vi "Confocal_Ver3.12f - sm correction.vi"() -> ()   [LabVIEW 2009]
uses:
  <vilib>/DAQmx/configure/timing.llb/DAQmx Timing (Sample Clock).vi
  <vilib>/DAQmx/create/channels.llb/DAQmx Create Channel (AI-Voltage-Basic).vi
  <vilib>/DAQmx/create/channels.llb/DAQmx Create Channel (AO-Voltage-Basic).vi
  <vilib>/DAQmx/write.llb/DAQmx Write (Analog 2D DBL NChan NSamp).vi
  <vilib>/DAQmx/read.llb/DAQmx Read (Analog 1D DBL NChan 1Samp).vi
  <vilib>/DAQmx/configure/trigger.llb/DAQmx Start Trigger (Digital Edge).vi
  <vilib>/DAQmx/read.llb/DAQmx Read (Analog 2D DBL NChan NSamp).vi
  <vilib>/DAQmx/write.llb/DAQmx Write (Analog 1D DBL NChan 1Samp).vi
  <vilib>/measure/NI_MABase.lvlib
  Program Files (x86)/National Instruments/LabVIEW 2009/resource/objmgr/daqmx.rc
panel:
  in  "Volts/pixel":dbl=0.1
  in  "Correction":dbl[][](array[numeric])=[[600.0, 650.0, 10.0, 5.0]]
  in  "sm correction?":bool
  out "Boolean":bool
  in  "Update":bool
  in  "StopPoint":dbl
  in  "Concat":bool
  in  "Increment":bool
  in  "stepsize":dbl=0.001
  in  "y 2":cluster{dbl, string, tag}[](array[cluster])=[{1.0, "", "Dev1/ai19"}, {1.0, "", "Dev1/ai16"}, {1.0, "", ""}, {1.0, "", ""}, {0.0, "", ""}, {1.0, "", ""}]
  in  "y":cluster{dbl, string, tag}[](array[cluster])=[{1.0, "", "Dev1/ao1"}, {1.0, "", "Dev1/ao0"}, {1.0, "", "Dev1/ao2"}, {1.0, "", "Dev1/ao3"}, {0.0, "", ""}, {1.0, "", ""}]
  in  "?":bool
  in  "Output4":dbl min=-10.0 max=10.0 step=0.1
  in  "Output3":dbl min=-10.0 max=10.0 step=0.1
  in  "Starting Point for Scan":tag="Dev1/ai1:2"
  in  "output scale":i32=1
  in  "out/in":dbl=1.0
  in  "Channel 2":path=path "T:/Physics/Minot Group/Lee/SPCM/2013-8-22/surf36_20"
  in  "Channel 1":path=path "T:/Physics/Minot Group/Lee/SPCM/2013-8-22/surf36_20"
  in  "Save Image":bool
  out "Channel2":dbl[][](graph)
  in  "Scanner delay (ms)":dbl=0.16
  in  "Lines read":u32=1
  out "Reflection Image":dbl[][](graph)
  out "Linescan":dbl[][](graph)=[[0.48392498883474516, 0.48650485009910055, 0.4823125755469766, 0.48553740212440066, 0.4842474714925252, 0.4852149194663185, 0.48392498883474516, 0.48263505820437946, 0.4813451275752202, 0.4813451275752202, 0.4813451275752202, 0.4787652663205165, 0.4823125755469766, 0.4748954744474811, 0.47650788772659863, 0.47586292241472655, 0.47618540507062507, 0.47586292241472655, 0.47715285303877103, 0.479732714290466, 0.4829575408618577, 0.48392498883474516, 0.48392498883474516, 0.4861823674407917, 0.48585988478255837, 0.4884397460505425, 0.4884397460505425, 0.48553740212440066, 0.48747229807448106, 0.4903746420047106, 0.4903746420047106, 0.4900521593454931, 0.4900521593454931, 0.4881172633917797, 0.4861823674407917, 0.4884397460505425, 0.4903746420047106, 0.4884397460505425, 0.4897296766863515, 0.4881172633917797, 0.48650485009910055, 0.48876222870938113, 0.4890847113682955, 0.4842474714925252, 0.4842474714925252, 0.4823125755469766, 0.4842474714925252, 0.4845699541503808, 0.4790877489770911, 0.4813451275752202, 0.479732714290466, 0.48070016226109263, 0.4800551969472663, 0.4784427836640171, 0.4803776796041418, 0.48166761023239696, 0.4832800235194114, 0.48166761023239696, 0.48102264491811875, 0.4852149194663185, 0.48650485009910055, 0.48585988478255837, 0.4877947807330925, 0.4871498154159452, 0.4894071940272856, 0.4881172633917797, 0.4871498154159452, 0.4900521593454931, 0.4877947807330925, 0.48747229807448106, 0.4861823674407917, 0.4848924368083119, 0.4832800235194114, 0.4871498154159452, 0.4871498154159452, 0.48553740212440066, 0.4868273327574851, 0.4852149194663185, 0.4852149194663185, 0.48263505820437946, 0.48166761023239696, 0.4800551969472663, 0.48102264491811875, 0.48392498883474516, 0.48070016226109263, 0.4787652663205165, 0.4748954744474811, 0.47457299179188256, 0.47296057851501405, 0.4736055438255367, 0.4703807172759168, 0.47747533569496986, 0.4842474714925252, 0.4997266391550764, 0.5158507723239795, 0.5342322843721873, 0.544229247171595, 0.573252687987951, 0.591634200841002, 0.6087257832047819, 0.6219475734938213, 0.6325895023644409, 0.6422639832349691, 0.6493586025881635, 0.6567757046830137, 0.6629028760126687, 0.6632253587150819, 0.6606454970981651, 0.6632253587150819, 0.6635478414175805, 0.6612904625018826, 0.6590330835903624, 0.6635478414175805, 0.6612904625018826, 0.6612904625018826, 0.6619354279059412, 0.6535508776797399, 0.6541958430797155, 0.650648533384047, 0.6516159814818486, 0.650648533384047, 0.6512934987824968, 0.6522609468808066, 0.6535508776797399, 0.6529059122801036, 0.6503260506849492, 0.6503260506849492, 0.6480686717936336, 0.6458112929064599, 0.6471012236986238, 0.6454888102086299, 0.6422639832349691, 0.6445213621156465, 0.6471012236986238, 0.6480686717936336, 0.650003567985936, 0.6535508776797399, 0.6545183257798305, 0.6538733603796852, 0.6535508776797399, 0.6551632911803154, 0.6561307392816795, 0.6600005316947886, 0.6622579106080984, 0.6587106008890573, 0.6606454970981651, 0.6577431527856528, 0.6587106008890573, 0.6580656354867026, 0.659678048993228, 0.6561307392816795, 0.6590330835903624, 0.6577431527856528, 0.6525834295804127, 0.6567757046830137, 0.6480686717936336, 0.6451663275108844, 0.6429089486290271, 0.6364592947035884, 0.6338794331428164, 0.6280747446506622, 0.6267848138783022, 0.6274297792643154, 0.6303321235055045, 0.6319445369757553, 0.63710426009462, 0.6387166735736678, 0.6409740524478638, 0.6474237063968759, 0.6496810852870074, 0.6532283949798794, 0.6529059122801036, 0.6529059122801036, 0.6538733603796852, 0.6538733603796852, 0.6541958430797155, 0.6545183257798305, 0.6554857738806851, 0.6570981873838084, 0.6593555662917526, 0.6606454970981651, 0.6616129452038693, 0.6658052203374621, 0.6632253587150819, 0.6616129452038693, 0.6622579106080984, 0.6645152895255886, 0.6570981873838084, 0.6567757046830137, 0.6525834295804127, 0.6483911544921392, 0.650648533384047, 0.6480686717936336, 0.6454888102086299, 0.6467787410004561, 0.6438763967207458, 0.6477461890952124, 0.650648533384047, 0.6461337756043742, 0.6512934987824968], [-0.0030237485169774024, -0.0030237485169774024, -0.0030237485169774024, -0.0030237485169774024, -0.003346231081005397, -0.0020563008246016422, -0.0036687136449847922, -0.0030237485169774024, -0.003346231081005397, -0.0030237485169774024, -0.0036687136449847922, -0.003346231081005397, -0.0030237485169774024, -0.00270126595290079, -0.0023787833887755428, -0.0036687136449847922, -0.003346231081005397, -0.0036687136449847922, -0.0036687136449847922, -0.003346231081005397, -0.003346231081005397, -0.0030237485169774024, -0.0036687136449847922, -0.0036687136449847922, -0.004313678772797855, -0.003991196208915606, -0.0030237485169774024, -0.0030237485169774024, -0.0036687136449847922, -0.003346231081005397, -0.003991196208915606, -0.0030237485169774024, -0.0030237485169774024, -0.003346231081005397, -0.003346231081005397, -0.0020563008246016422, -0.00270126595290079, -0.0020563008246016422, -0.0020563008246016422, -0.0020563008246016422, -0.0030237485169774024, -0.00270126595290079, -0.003346231081005397, -0.00270126595290079, -0.0030237485169774024, -0.0036687136449847922, -0.0036687136449847922, -0.003991196208915606, -0.0030237485169774024, -0.0036687136449847922, -0.0023787833887755428, -0.0030237485169774024, -0.00270126595290079, -0.003346231081005397, -0.00270126595290079, -0.00270126595290079, -0.0030237485169774024, -0.00270126595290079, -0.003991196208915606, -0.0036687136449847922, -0.003346231081005397, -0.0030237485169774024, -0.003991196208915606, -0.003346231081005397, -0.0036687136449847922, -0.003346231081005397, -0.00270126595290079, -0.0036687136449847922, -0.0030237485169774024, -0.0036687136449847922, -0.003346231081005397, -0.003346231081005397, -0.0036687136449847922, -0.003991196208915606, -0.0036687136449847922, -0.0036687136449847922, -0.003346231081005397, -0.0036687136449847922, -0.0036687136449847922, -0.003991196208915606, -0.0036687136449847922, -0.0030237485169774024, -0.0036687136449847922, -0.00270126595290079, -0.004313678772797855, -0.004958643900416732, -0.0065710567186153, -0.0068935392821096765, -0.008505952098855858, -0.008828434662060078, -0.010118364914394162, -0.01108581260313829, -0.010440847477357074, -0.008183469535603323, -0.005603609027841567, -0.00270126595290079, 0.0014910073845274476, 0.00858562382054782, 0.013422862313310125, 0.018905065951914643, 0.022774856764300203, 0.027289612721192864, 0.030836920979949438, 0.03180436868794224, 0.03277181639638989, 0.03277181639638989, 0.03180436868794224, 0.030836920979949438, 0.02890202556532645, 0.026322165015316323, 0.024709752173193242, 0.02180740906052947, 0.02051747878953489, 0.019227548519338968, 0.016647687981338526, 0.01568024028040894, 0.014712792579926194, 0.01277789718029931, 0.01277789718029931, 0.011487966914871401, 0.00955307151821172, 0.00858562382054782, 0.007940658689018203, 0.006973210992092902, 0.00600576329561012, 0.006328245861055242, 0.005683280730214114, 0.005360798164867205, 0.005038315599569377, 0.004070867903970193, 0.00471583303432061, 0.004070867903970193, 0.0031034202088120865, 0.0027809376438573193, 0.0018134899492865714, 0.0014910073845274476, 0.0014910073845274476, 0.0021359725140945793, 0.0014910073845274476, 0.0008460422551557815, 0.00020107712597943893, 0.0005235596905432037, -0.0004438880030017225, -0.0004438880030017225, -0.0004438880030017225, -0.0007663705674191548, -0.0007663705674191548, -0.001088853131787845, -0.0014113356961078113, -0.001733818260379071, -0.0023787833887755428, -0.001733818260379071, -0.0023787833887755428, -0.001733818260379071, -0.0023787833887755428, -0.0023787833887755428, -0.0020563008246016422, -0.00270126595290079, -0.0023787833887755428, -0.0020563008246016422, -0.00270126595290079, -0.00270126595290079, -0.0023787833887755428, -0.001733818260379071, -0.0014113356961078113, -0.001733818260379071, -0.0023787833887755428, -0.0023787833887755428, -0.0023787833887755428, -0.0023787833887755428, -0.00270126595290079, -0.0020563008246016422, -0.003346231081005397, -0.0023787833887755428, -0.00270126595290079, -0.00270126595290079, -0.0020563008246016422, -0.0030237485169774024, -0.0023787833887755428, -0.0030237485169774024, -0.0020563008246016422, -0.003346231081005397, -0.0023787833887755428, -0.00270126595290079, -0.0030237485169774024, -0.0020563008246016422, -0.003346231081005397, -0.003346231081005397, -0.003991196208915606, -0.003346231081005397, -0.00270126595290079, -0.0030237485169774024, -0.0036687136449847922, -0.00270126595290079, -0.0023787833887755428, -0.00270126595290079, -0.003991196208915606, -0.0036687136449847922, -0.003346231081005397, -0.00270126595290079]]
  out "Output rate":dbl=31250.0
  out "Input rate":dbl=31250.0
  in  "Y Scan size(um)":dbl=2.0
  in  "Reset":bool
  in  "Stop":bool
  in  "Continuous \nScan":bool=TRUE
  in  "Finite scan":bool
  in  "Conversion \n(mV/um)":dbl=41.0
  in  "Scan Lines":u32=200
  in  "Scan Points":u32=200
  in  "Scan Angle (degrees)":dbl
  in  "X offset (um)":dbl=-0.4599999999999997
  in  "Y offset (um)":dbl=-0.23
  in  "Scan Rate (Hz)":dbl=25.0
  in  "X Scan size(um)":dbl=2.0
  in  "minimum value":dbl=-4.0 caption="Output Minimum Value" format="%0.2f"
  in  "maximum value":dbl=4.0 caption="Output Maximum Value" format="%0.2f"
  in  "Maximum Value":dbl=10.0 caption="Input Maximum Value" format="%0.2f"
  in  "Minimum Value":dbl=-10.0 caption="Input Minimum Value" format="%0.2f"
  # "Scan channel 1"
  # "Scan channel 2"
  # "Device"
  # "Output channel 3"
  # "Output channel 4"
  # "Input channel 1"
  # "Input channel 2"
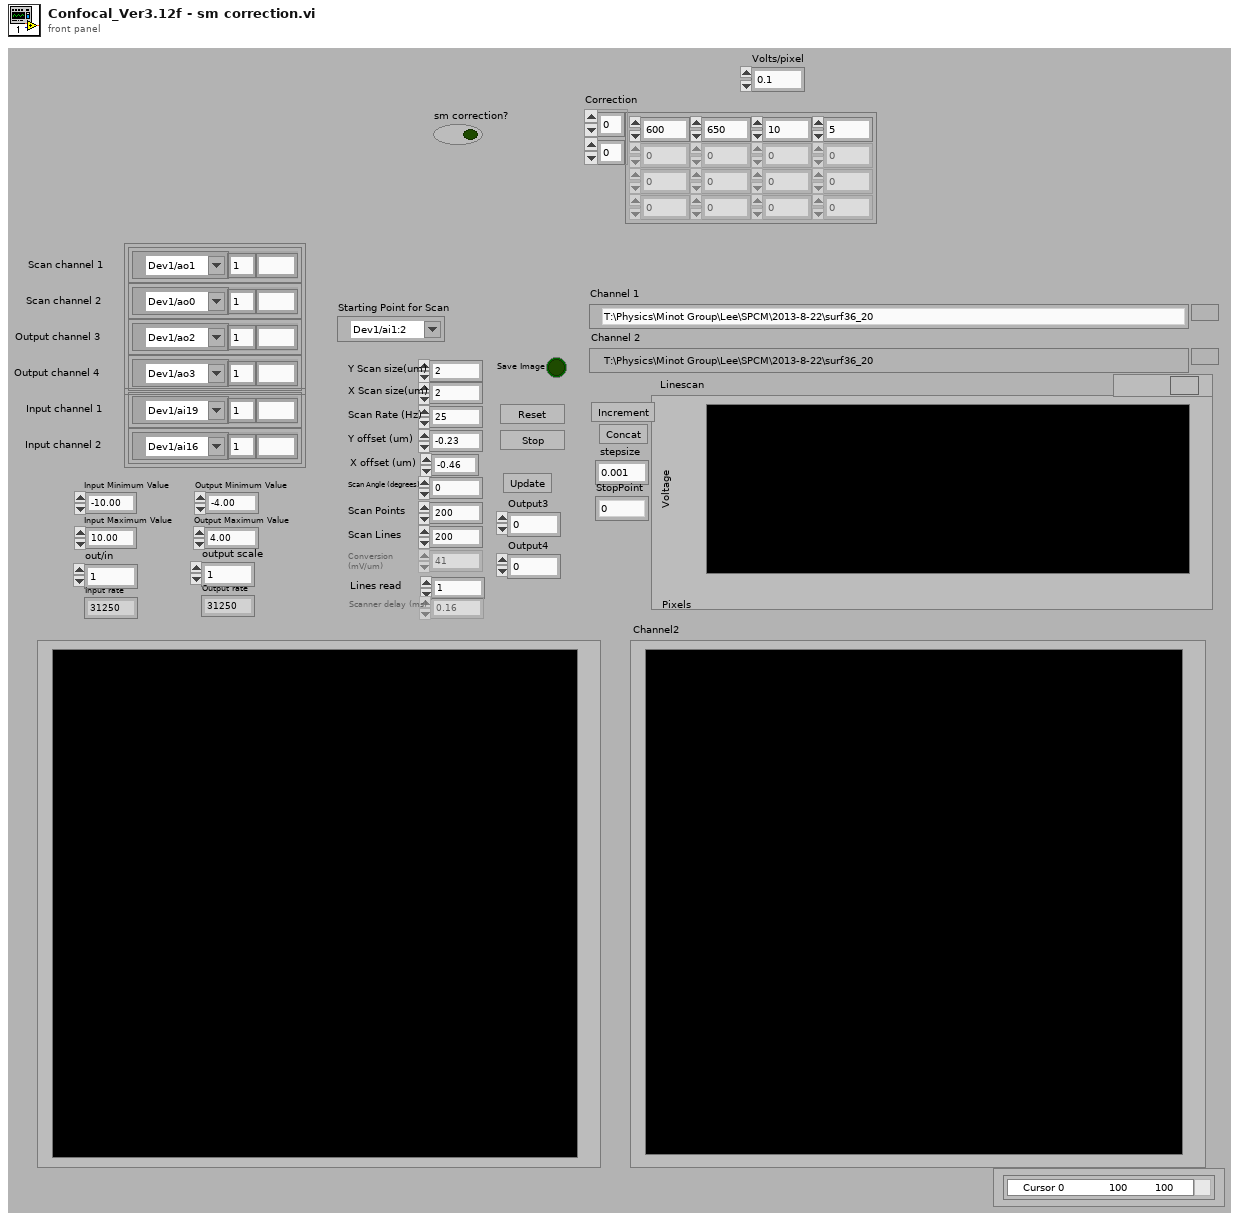
[diagram p1: front panel]
types:
  T1 = enum16{"Sine Wave", "Triangle Wave", "Square Wave", "Sawtooth Wave"}
  T2 = cluster{"Y Scan size(um) ":dbl, "X Scan size(um)":dbl, "Scan Rate (Hz)":dbl, "Y offset (um)":dbl, "X offset (um)":dbl, "Scan Angle (degrees)":dbl, "Scan Points":u32, "Scan Lines":u32, "Conversion \n(mV/um)":dbl, "Finite scan":bool, "Continuous \nScan":bool, "Lines read":u32, "Scanner delay (ms)":dbl}
  T3 = enum16{"open", "open or create", "create or replace", "create", "open (read only)"}
  T4 = typedef "LVPointDoubleTypeDef.ctl" = cluster{"Cursor X":dbl, "Cursor Y":dbl}
  T5 = cluster{"X offset (um)":dbl, "Y offset (um)":dbl}
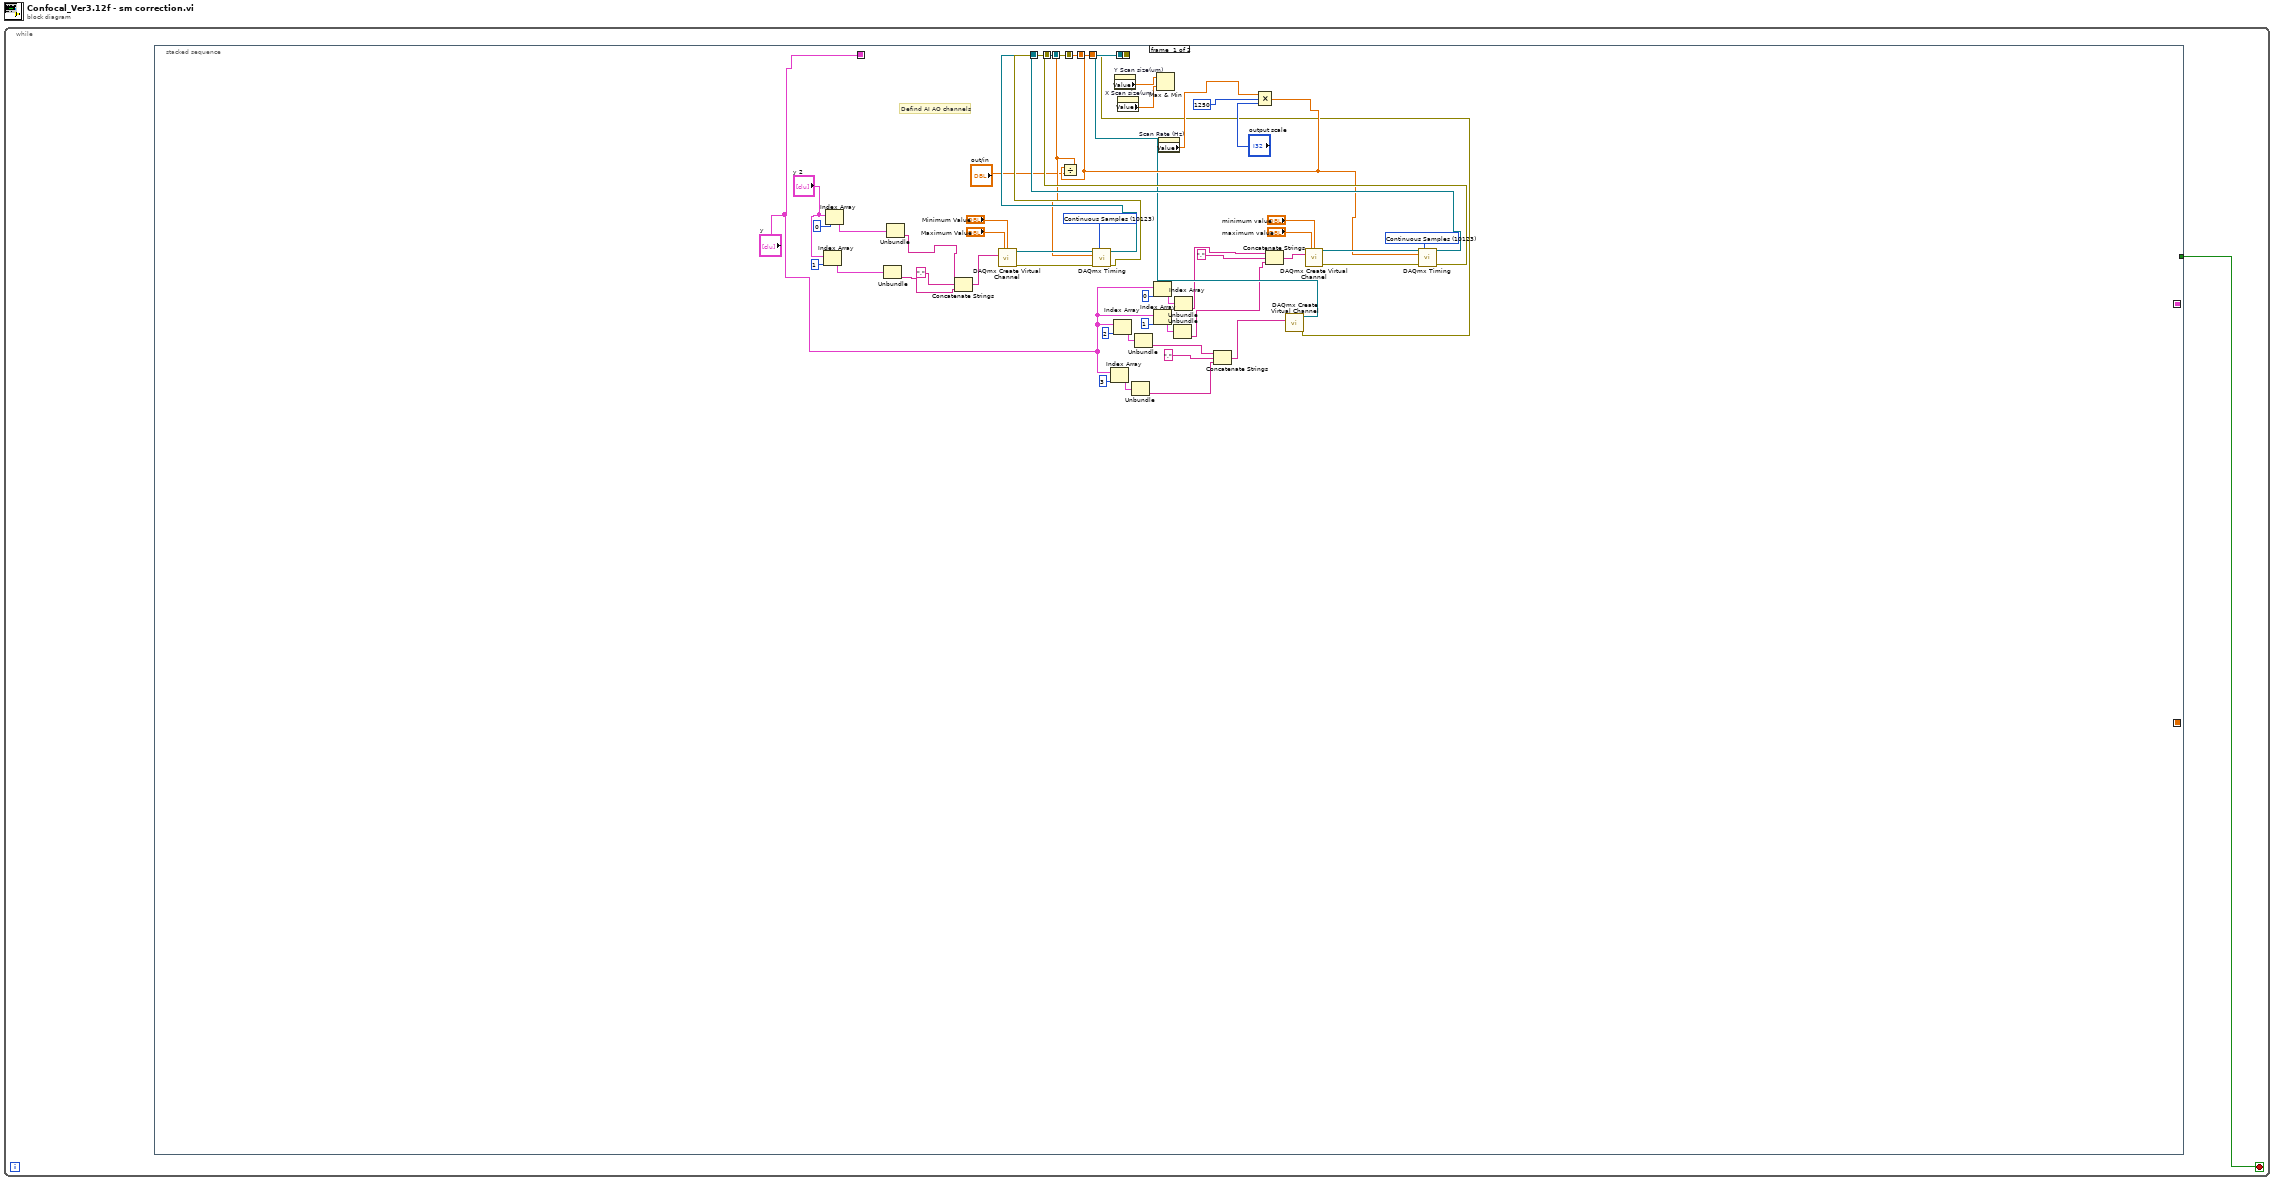
[diagram p0: block diagram]
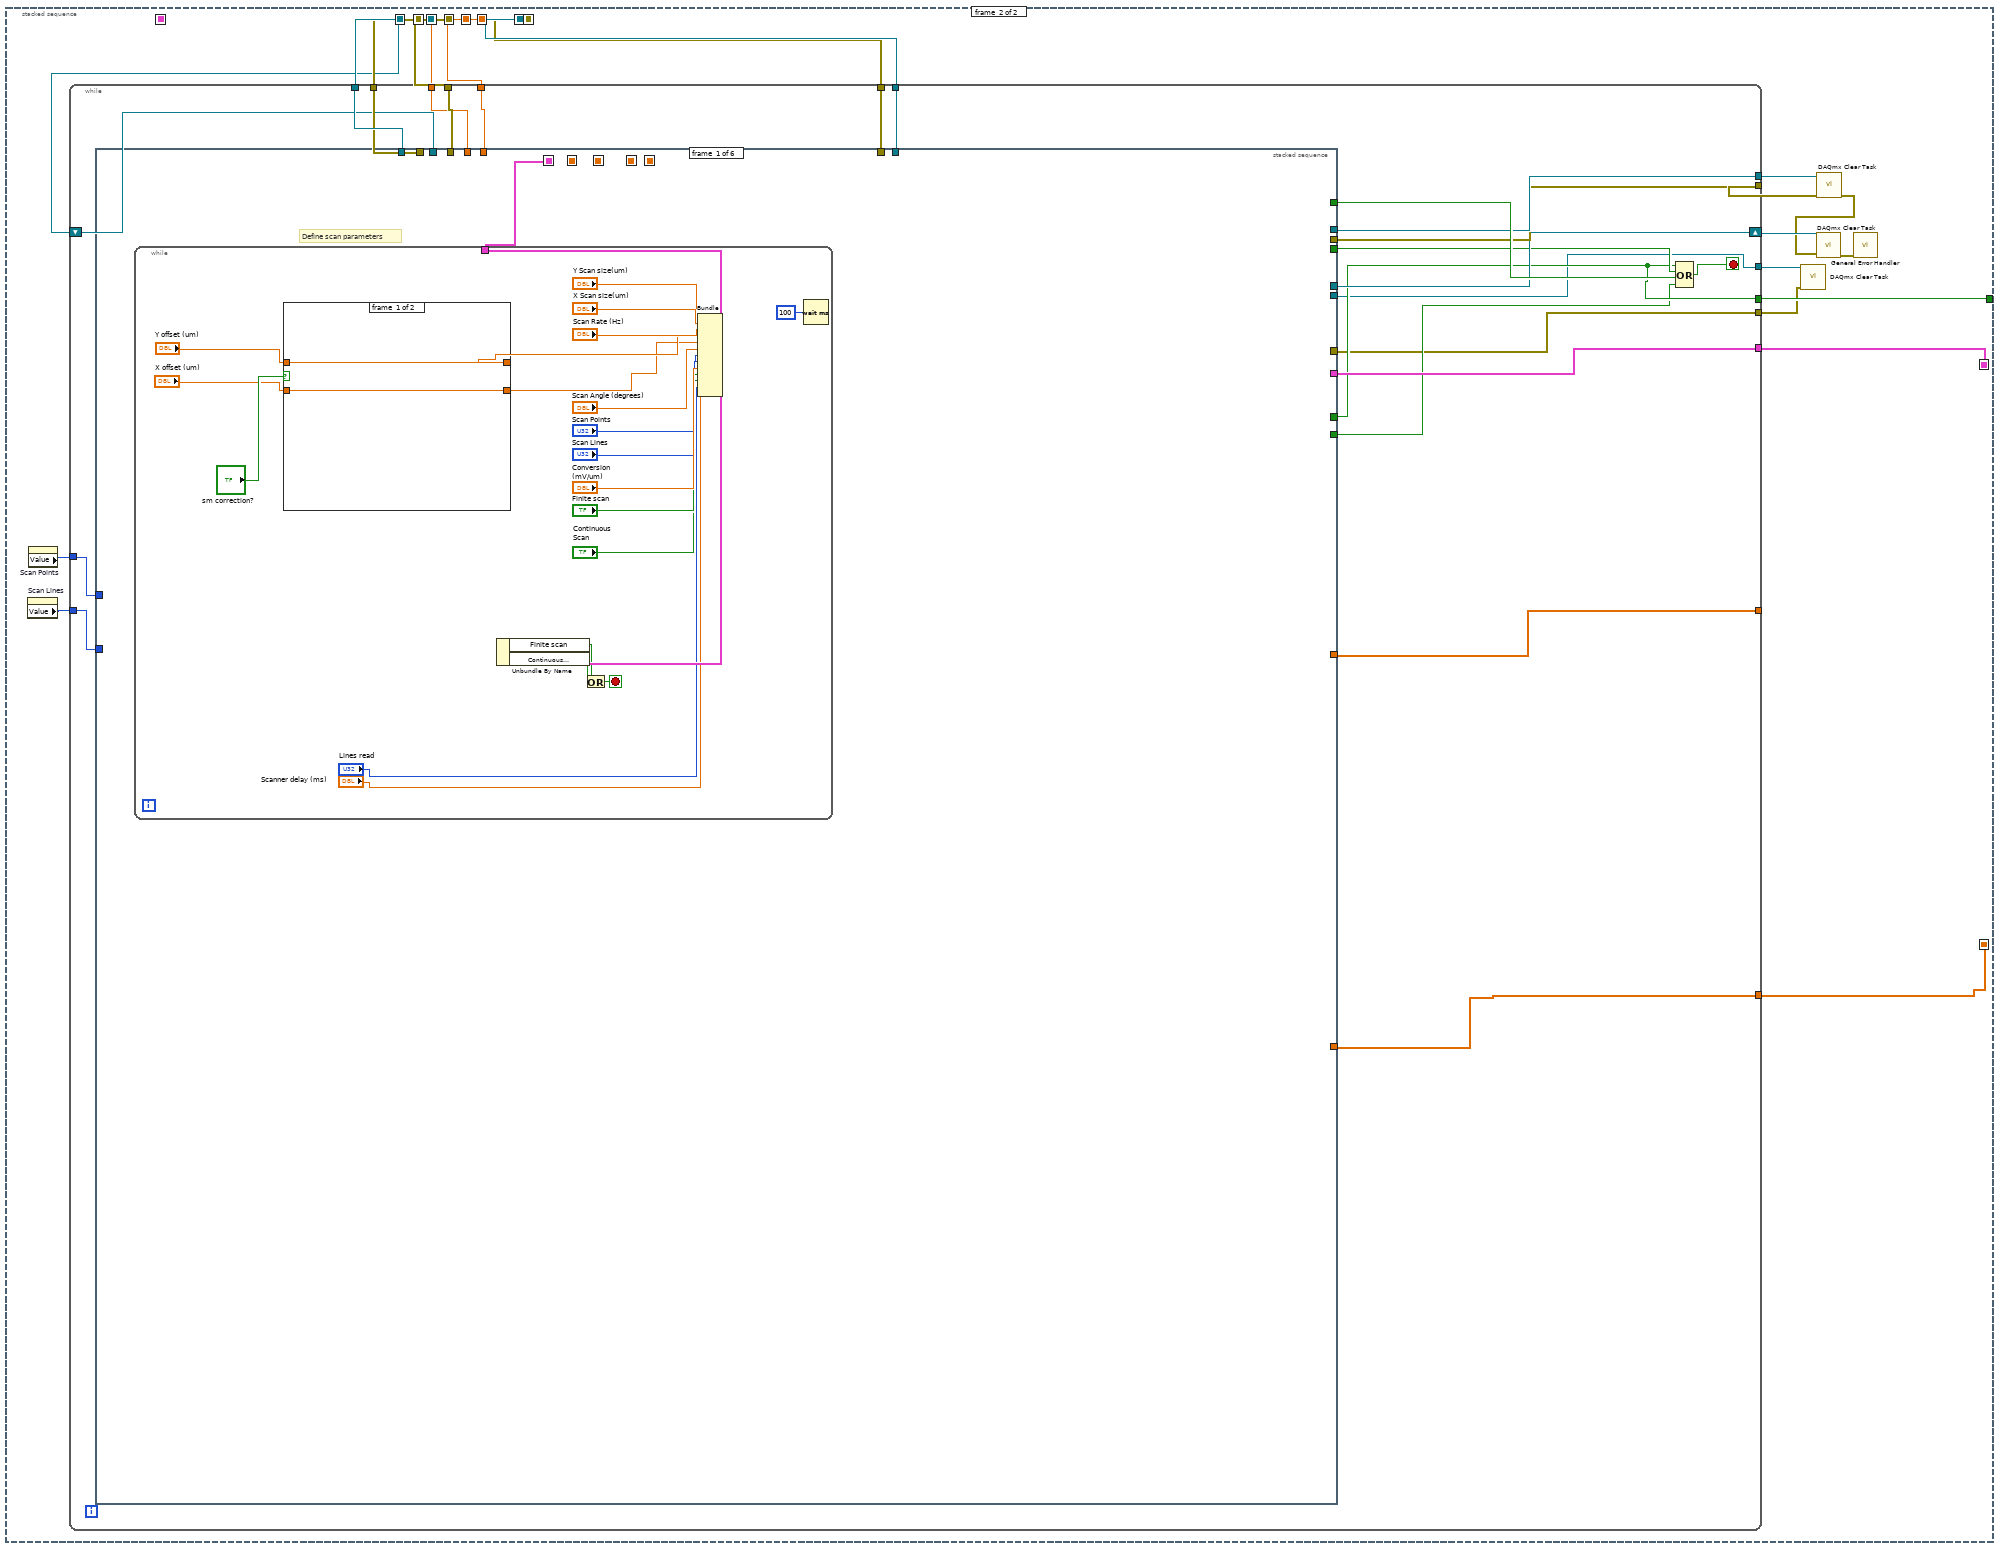
[diagram p2: hidden frame]
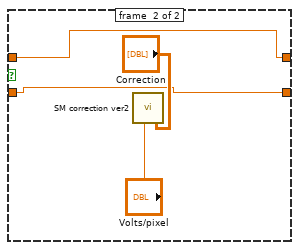
[diagram p3: hidden frame]
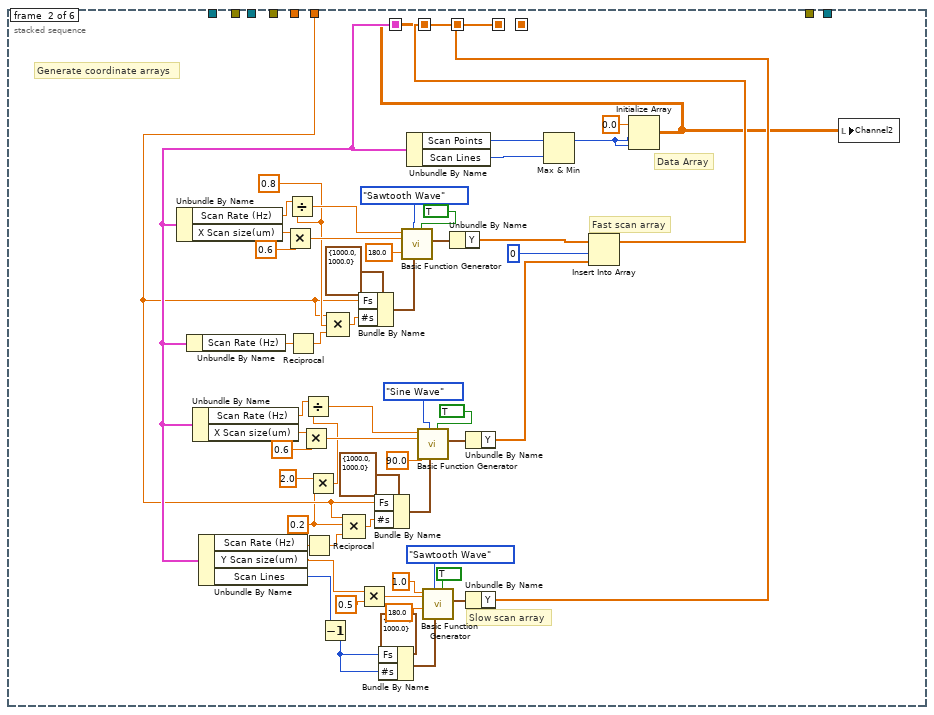
[diagram p4: hidden frame]
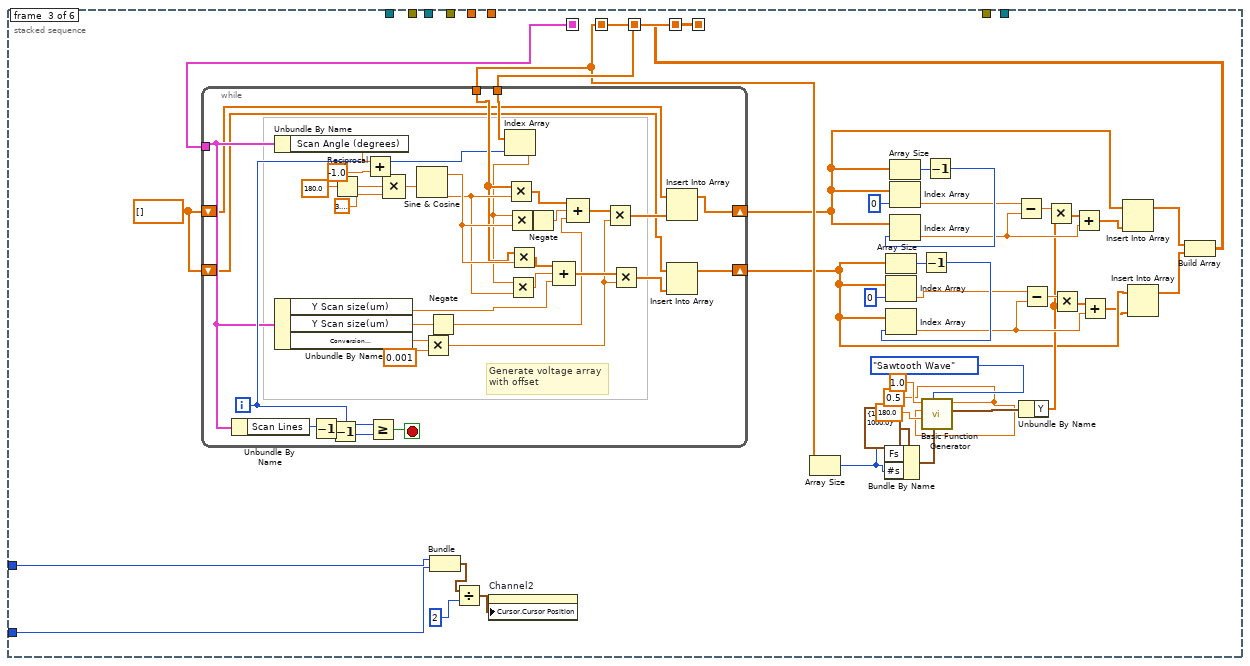
[diagram p5: hidden frame]
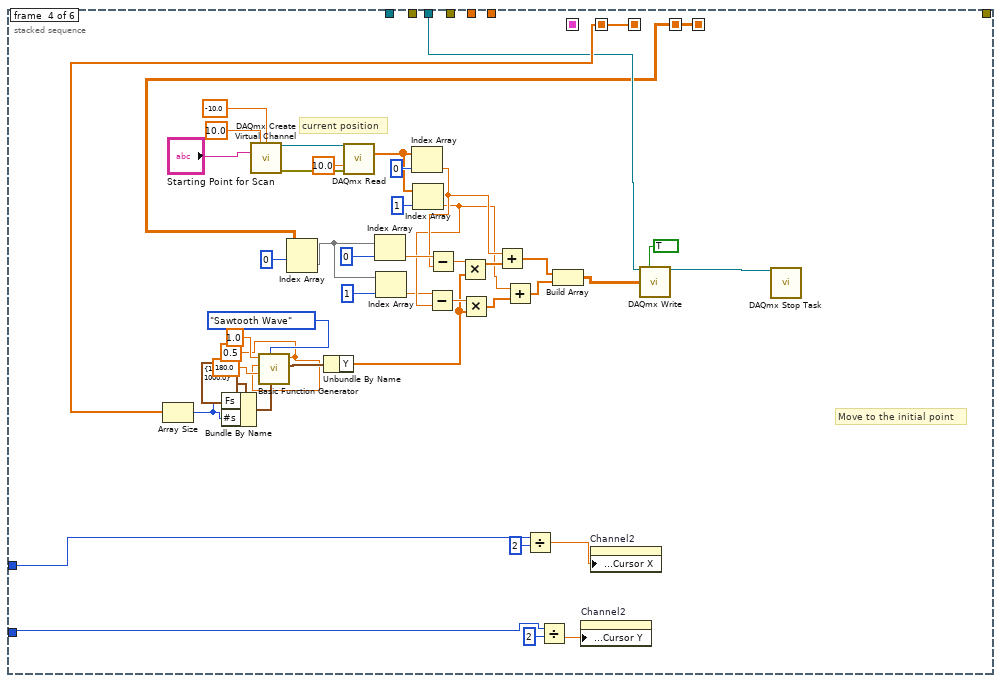
[diagram p6: hidden frame]
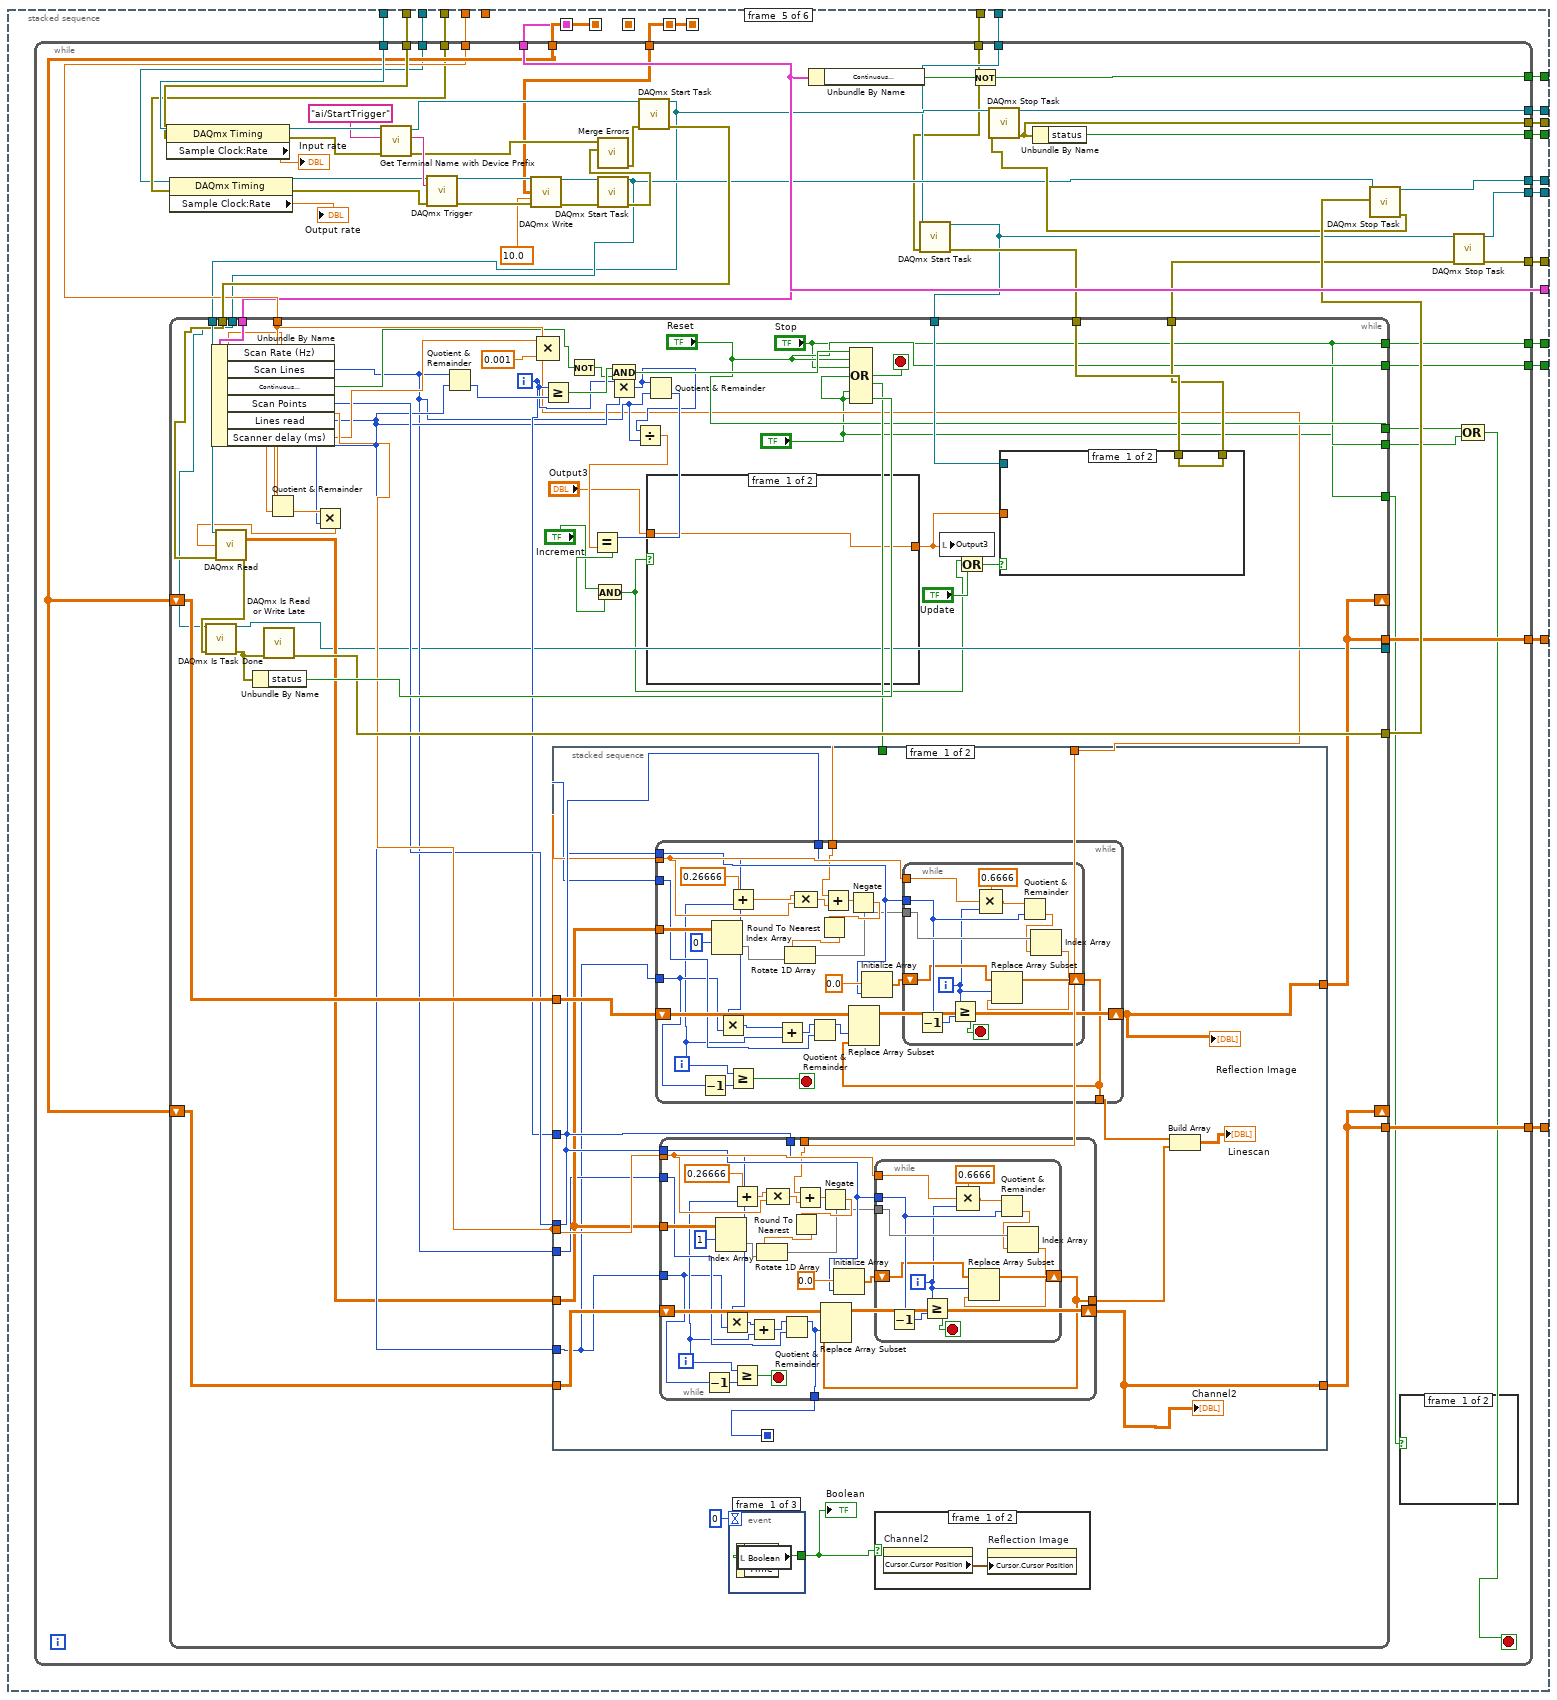
[diagram p7: hidden frame]
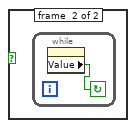
[diagram p8: hidden frame]
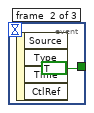
[diagram p9: hidden frame]
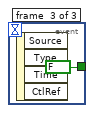
[diagram p10: hidden frame]
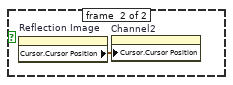
[diagram p11: hidden frame]
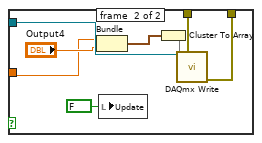
[diagram p12: hidden frame]
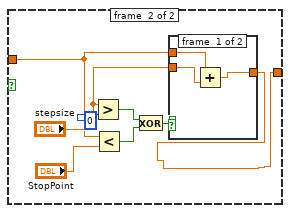
[diagram p13: hidden frame]
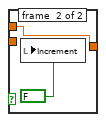
[diagram p14: hidden frame]
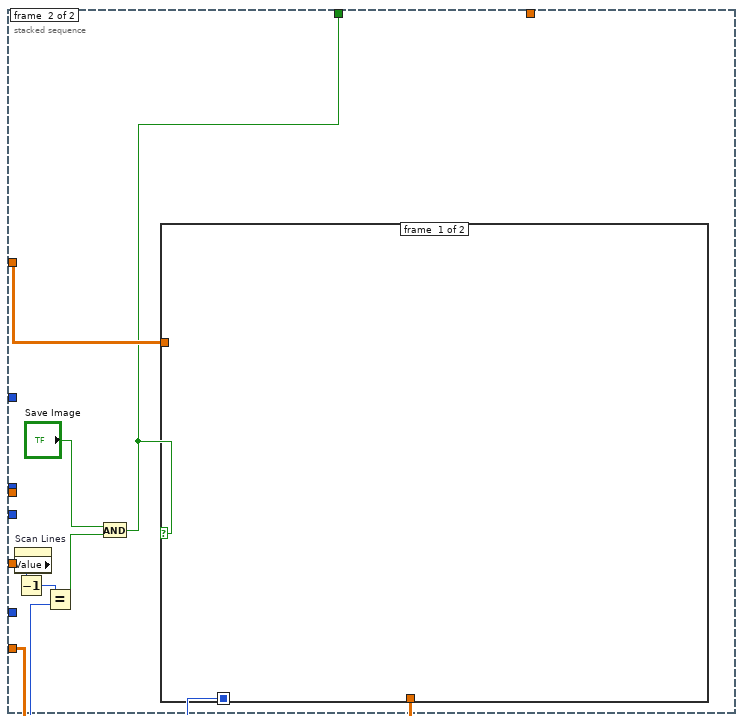
[diagram p15: hidden frame]
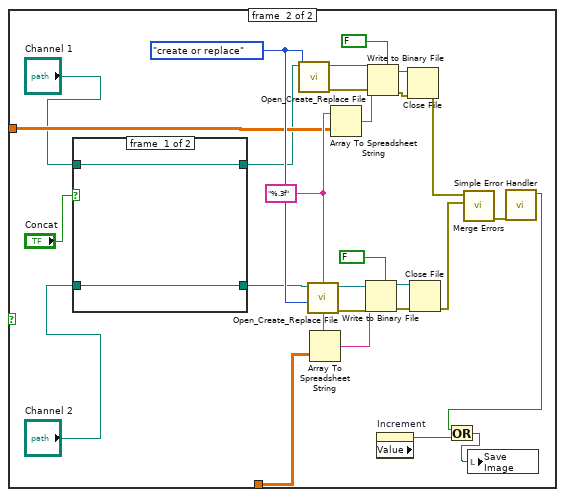
[diagram p16: hidden frame]
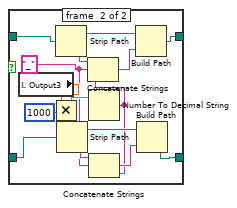
[diagram p17: hidden frame]
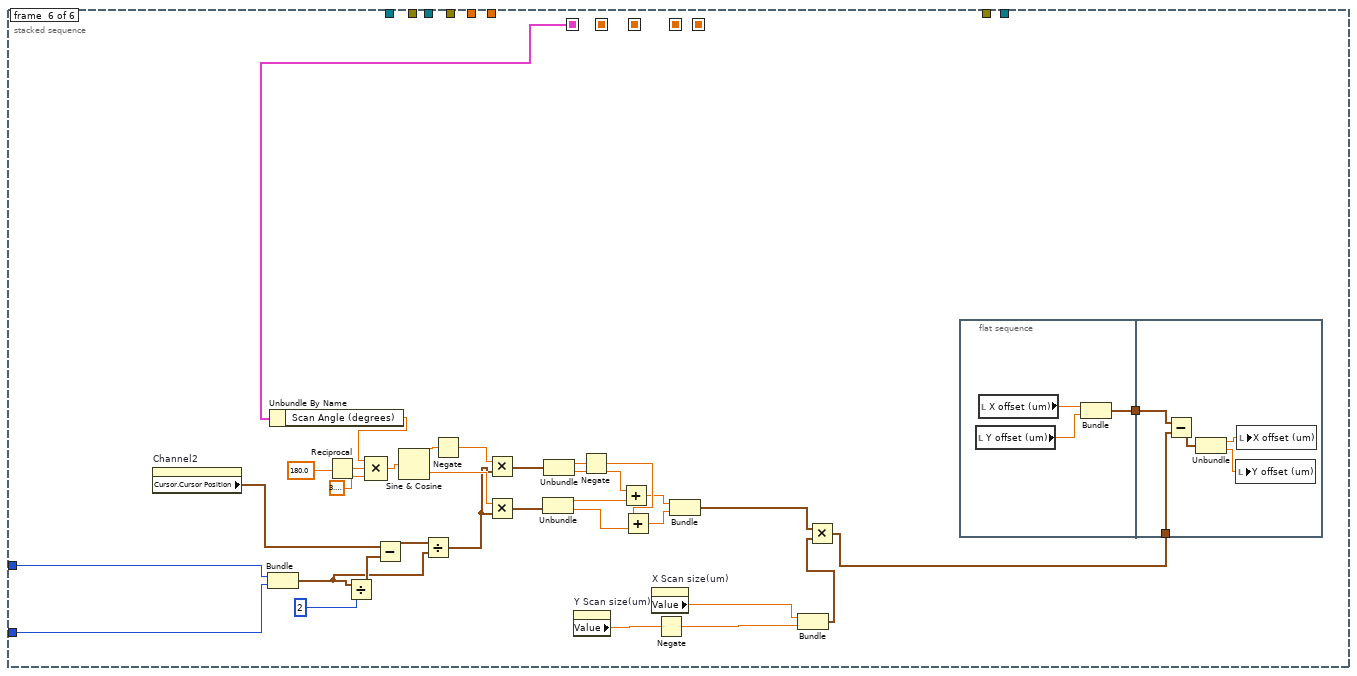
[diagram p18: hidden frame]
diagram:
  n1 = while {
    stop <- w1 stop-if-true
    n2 = stacked-sequence {
      seq-local: [w39 _] -> [_ w70]
      seq-local: [w42 _] -> [_ w69]
      seq-local: [w41 _] -> [_ w62]
      seq-local: [w40 _] -> [_ w68]
      seq-local: [w34 _] -> [_ w67]
      seq-local: [w33 _] -> [_ w71]
      seq-local: [_ w61] -> [_ _]
      seq-local: [_ w60] -> [_ _]
      seq-local: [w29 _] -> [_ w56]
      seq-local: [w28 _] -> [_ w55]
      seq-local: ["y" _] -> [_ _]
      tunnel: [_ w57] -> w1
      frame #0 {
        w44 = 10123 items=["Finite Samples"=10178, "Continuous Samples"=10123] ("sample mode")
        w49 = 10123 items=["Finite Samples"=10178, "Continuous Samples"=10123] ("sample mode")
        # "Defind AI AO channels"
        n3 = Index Array(array="y 2", index=1) -> (element=w20:cluster{dbl, string, tag})
        n4 = Index Array(array="y 2", index=0) -> (element=w22:cluster{dbl, string, tag})
        n5 = Unbundle(w20) -> (w2:tag)  [unwired: 2 out]
        n6 = Unbundle(w22) -> (w3:tag)  [unwired: 2 out]
        n7 = Concatenate Strings(w3, ",", w2) -> (w27:string)
        n8 = call-poly <vilib>:"DAQmx Create Virtual Channel.vi"("maximum value"="Maximum Value", "minimum value"="Minimum Value", "physical channels"=w27) -> ("task out"=w47:refnum<k21>, "error out"=w48:errorcluster)  [unwired: 11 in]
        n9 = Index Array(array="y", index=3) -> (element=w15:cluster{dbl, string, tag})
        n10 = Index Array(array="y", index=2) -> (element=w17:cluster{dbl, string, tag})
        n11 = property on="Y Scan size(um)" class="Digital (strict)"() -> ("Value"=w36:dbl)  [unwired: 2 in, 2 out]
        n12 = property on="X Scan size(um)" class="Digital (strict)"() -> ("Value"=w35:dbl)  [unwired: 2 in, 2 out]
        n13 = Unbundle(w15) -> (w13:tag)  [unwired: 2 out]
        n14 = Unbundle(w17) -> (w14:tag)  [unwired: 2 out]
        n15 = Index Array(array="y", index=1) -> (element=w9:cluster{dbl, string, tag})
        n16 = Index Array(array="y", index=0) -> (element=w11:cluster{dbl, string, tag})
        n17 = Max & Min(x=w36, y=w35) -> ()  [unwired: 2 out]
        n18 = property on="Scan Rate (Hz)" class="Digital (strict)"() -> ("Value"=w31:dbl)  [unwired: 2 in, 2 out]
        n19 = Unbundle(w9) -> (w7:tag)  [unwired: 2 out]
        n20 = Unbundle(w11) -> (w8:tag)  [unwired: 2 out]
        n21 = Concatenate Strings(w14, ",", w13) -> (w4:string)
        n22 = Compound Arithmetic op=MULTIPLY(w31, 1250, "output scale") -> (w33:dbl)
        n23 = Divide(x=w33, y="out/in") -> (x/y=w34:dbl)
        n24 = call-poly <vilib>:"DAQmx Timing.vi"("task/channels in"=w47, "sample mode"=w49, "rate"=w34, "error in"=w48) -> ("task out"=w39:refnum<k21>, "error out"=w42:errorcluster)  [unwired: 10 in]
        n25 = Concatenate Strings(w8, ",", w7) -> (w24:string)
        n26 = call-poly <vilib>:"DAQmx Create Virtual Channel.vi"("physical channels"=w4) -> ("task out"=w29:refnum<k21>, "error out"=w28:errorcluster)  [unwired: 13 in]
        n27 = call-poly <vilib>:"DAQmx Create Virtual Channel.vi"("maximum value"="maximum value", "minimum value"="minimum value", "physical channels"=w24) -> ("task out"=w38:refnum<k21>, "error out"=w43:errorcluster)  [unwired: 11 in]
        n28 = call-poly <vilib>:"DAQmx Timing.vi"("task/channels in"=w38, "sample mode"=w44, "rate"=w33, "error in"=w43) -> ("task out"=w41:refnum<k21>, "error out"=w40:errorcluster)  [unwired: 10 in]
      }
      frame #1 {
        n29 = property on="Scan Lines" class="Digital (strict)"() -> ("Value"=w59:u32)  [unwired: 2 in, 2 out]
        n30 = property on="Scan Points" class="Digital (strict)"() -> ("Value"=w58:u32)  [unwired: 2 in, 2 out]
        n31 = while {
          tunnel: w71 -> [w94]
          tunnel: w70 -> [w93]
          tunnel: w69 -> [w92]
          tunnel: w68 -> [w91]
          tunnel: w67 -> [w90]
          tunnel: [w88] -> w66
          tunnel: [w87] -> w65
          shift-right: [w85] -> w64
          shift-left: w62 -> [w84]
          tunnel: [w83] -> _
          tunnel: [w82] -> w61
          tunnel: [w80] -> w60
          tunnel: w59 -> [w79]
          tunnel: w58 -> [w78]
          tunnel: [w77] -> w57
          tunnel: w56 -> [w75]
          tunnel: w55 -> [w74]
          tunnel: [w73] -> w53
          tunnel: [w72] -> w52
          stop <- w86 stop-if-true
          n32 = stacked-sequence {
            seq-local: [w95 _ _ _ _ _] -> [_ w148 w216 _ w304 w621]
            seq-local: [_ w123 _ _ _ _] -> [_ _ _ _ w311 _]
            seq-local: [_ w124 _ _ _ _] -> [_ _ w206 w265 _ _]
            seq-local: [_ w125 _ _ _ _] -> [_ _ w217 _ _ _]
            seq-local: [_ _ w179 _ _ _] -> [_ _ _ w261 w308 _]
            tunnel: w94 -> [_ w147 _ _ _ _]
            tunnel: w93 -> [_ _ _ _ w319 _]
            tunnel: w92 -> [_ _ _ _ w318 _]
            tunnel: w84 -> [_ _ _ w263 w307 _]
            tunnel: w91 -> [_ _ _ _ w317 _]
            tunnel: w90 -> [_ _ _ _ w309 _]
            tunnel: [_ _ _ _ w316 _] -> w77
            tunnel: [_ _ _ _ w315 _] -> w81
            tunnel: [_ _ _ _ w310 _] -> w89
            tunnel: [_ _ _ _ w314 _] -> w88
            tunnel: [_ _ _ _ w313 _] -> w87
            tunnel: [_ _ _ _ w312 _] -> w85
            tunnel: [_ _ _ _ w306 _] -> w83
            tunnel: [_ _ _ _ w305 _] -> w82
            tunnel: [_ _ _ _ w304 _] -> w80
            tunnel: [_ _ _ _ w303 _] -> w76
            tunnel: w79 -> [_ _ w181 w255 _ w596]
            tunnel: w78 -> [_ _ w182 w256 _ w595]
            tunnel: w75 -> [_ _ _ _ w302 _]
            tunnel: w74 -> [_ _ _ _ w301 _]
            tunnel: [_ _ _ _ w300 _] -> w73
            tunnel: [_ _ _ _ w299 _] -> w72
            frame #0 {
              # "Define scan parameters"
              n33 = while {
                tunnel: [w110] -> w95
                stop <- w111 stop-if-true
                n34 = case shown="True" "sm correction?" {
                  tunnel: [w118 w120] -> w99
                  tunnel: "Y offset (um)" -> [w118 w120]
                  tunnel: [w117 w119] -> w97
                  tunnel: "X offset (um)" -> [w117 w119]
                  frame #0 {
                  }
                  frame #1 {
                    n35 = call "SM correction ver2.vi"("Volts/pixel"="Volts/pixel", "Array"="Correction") -> ()  [unwired: 5 in, 2 out]
                  }
                }
                n36 = Bundle("Y Scan size(um)"="Y Scan size(um)", "X Scan size(um)"="X Scan size(um)", "Scan Rate (Hz)"="Scan Rate (Hz)", "Y offset (um)"=w99, "X offset (um)"=w97, "Scan Angle (degrees)"="Scan Angle (degrees)", "Scan Points"="Scan Points", "Scan Lines"="Scan Lines", "Conversion \n(mV/um)"="Conversion \n(mV/um)", "Finite scan"="Finite scan", "Continuous \nScan"="Continuous \nScan", "Lines read"="Lines read", "Scanner delay (ms)"="Scanner delay (ms)") -> (w110:T2)  [unwired: 1 in]
                n37 = Unbundle By Name(w110) -> ("Finite scan"=w109:bool, "Continuous \nScan"=w108:bool)
                n38 = Or(x=w109, y=w108) -> (x .or. y?=w111:bool)
                n39 = Wait (ms)(milliseconds to wait=u32 100) -> ()  [unwired: 1 out]
              }
            }
            frame #1 {
              w127 = 0.2 ("value")
              w166 = 0.8 ("y")
              # "Slow scan array"
              # "Fast scan array"
              # "Data Array"
              # "Generate coordinate arrays"
              n40 = Unbundle By Name(w148) -> ("Scan Rate (Hz)"=w171:dbl, "X Scan size(um)"=w174:dbl)
              n41 = Unbundle By Name(w148) -> ("Scan Rate (Hz)"=w164:dbl)
              n42 = Unbundle By Name(w148) -> ("Scan Rate (Hz)"=w156:dbl, "X Scan size(um)"=w159:dbl)
              n43 = Unbundle By Name(w148) -> ("Scan Rate (Hz)"=w150:dbl, "Y Scan size(um)"=w139:dbl, "Scan Lines"=w140:u32)
              n44 = Multiply(x=w174, y=0.6) -> (x*y=w172:dbl)
              n45 = Divide(x=w171, y=w166) -> (x/y=w170:dbl)
              n46 = Reciprocal(x=w164) -> (1/x=w165:dbl)
              n47 = Multiply(x=w159, y=0.6) -> (x*y=w157:dbl)
              n48 = Reciprocal(x=w150) -> (1/x=w151:dbl)
              n49 = Multiply(x=2.0, y=w127) -> (x*y=w126:dbl)
              n50 = Divide(x=w156, y=w126) -> (x/y=w155:dbl)
              n51 = Decrement(x=w140) -> (x-1=w132:u32)
              n52 = Compound Arithmetic op=MULTIPLY(w147, w166, w165) -> (w167:dbl)
              n53 = Compound Arithmetic op=MULTIPLY(w147, w127, w151) -> (w152:dbl)
              n54 = Bundle By Name(cluster=cluster{"Fs":dbl, "#s":dbl} {"Fs"=1000.0, "#s"=1000.0} ("sampling info"), "Fs"=w147, "#s"=w167) -> (w168:cluster{"Fs":dbl, "#s":dbl})
              n55 = Multiply(x=w139, y=0.5) -> (x*y=w138:dbl)
              n56 = Bundle By Name(cluster=cluster{"Fs":dbl, "#s":dbl} {"Fs"=1000.0, "#s"=1000.0} ("sampling info"), "Fs"=w147, "#s"=w152) -> (w153:cluster{"Fs":dbl, "#s":dbl})
              n57 = Bundle By Name(cluster=cluster{"Fs":dbl, "#s":dbl} {"Fs"=1000.0, "#s"=1000.0} ("sampling info"), "Fs"=w132, "#s"=w132) -> (w141:cluster{"Fs":dbl, "#s":dbl})
              n58 = call <vilib>:"Basic Function Generator.vi"("reset signal"=TRUE, "sampling info"=w168, "signal type"=T1."Sawtooth Wave", "phase"=180.0, "amplitude"=w172, "frequency"=w170) -> ("signal out"=w163:waveform(dbl))  [unwired: 3 in, 2 out]
              n59 = Unbundle By Name(w148) -> ("Scan Points"=w131:u32, "Scan Lines"=w130:u32)
              n60 = call <vilib>:"Basic Function Generator.vi"("reset signal"=TRUE, "sampling info"=w153, "signal type"=T1."Sine Wave", "phase"=90.0, "amplitude"=w157, "frequency"=w155) -> ("signal out"=w149:waveform(dbl))  [unwired: 3 in, 2 out]
              n61 = call <vilib>:"Basic Function Generator.vi"("reset signal"=TRUE, "sampling info"=w141, "signal type"=T1."Sawtooth Wave", "phase"=180.0, "amplitude"=w138, "frequency"=1.0) -> ("signal out"=w134:waveform(dbl))  [unwired: 3 in, 2 out]
              n62 = Unbundle By Name(w163) -> ("Y"=w136:dbl[])
              n63 = Unbundle By Name(w149) -> ("Y"=w146:dbl[])
              n64 = Unbundle By Name(w134) -> ("Y"=w125:dbl[])
              n65 = Max & Min(x=w131, y=w130) -> (max(x,y)=w129:u32)  [unwired: 1 out]
              n66 = Insert Into Array(array=w136, index=0, new element=w146) -> (w124:dbl[])
              n67 = Initialize Array(0.0 ("element"), w129, w129) -> (w123:dbl[][])
              n68 = local write "Channel2"(w123) -> ()
            }
            frame #2 {
              w208 = 0.5 ("offset")
              w215 = dbl[] []
              n69 = while {
                tunnel: w216 -> [w237]
                tunnel: w206 -> [w243]
                tunnel: w217 -> [w242]
                shift-right: [w229] -> w188
                shift-left: w215 -> [w228]
                shift-right: [w225] -> w189
                shift-left: w215 -> [w226]
                i -> [w240]
                stop <- w234 stop-if-true
                # "Generate voltage array\nwith offset"
                n70 = Unbundle By Name(w237) -> ("Scan Lines"=w239:u32)
                n71 = Unbundle By Name(w237) -> ("Scan Angle (degrees)"=w253:dbl)
                n72 = Unbundle By Name(w237) -> ("Y Scan size(um)"=w218:dbl, "Y Scan size(um)"=w220:dbl, "Conversion \n(mV/um)"=w236:dbl)
                n73 = Decrement(x=w239) -> (x-1=w238:u32)
                n74 = Decrement(x=w238) -> (x-1=w224:u32)
                n75 = Reciprocal(x=180.0 ("value")) -> (1/x=w252:dbl)
                n76 = Add(x=w253, y=-1.0) -> (x+y=w223:dbl)
                n77 = Greater Or Equal?(x=w240, y=w224) -> (x >= y?=w234:bool)
                n78 = Compound Arithmetic op=MULTIPLY(w223, w252, 3.141592653589793) -> (w254:dbl)
                n79 = Sine & Cosine(0:w254) -> (1:w250:dbl, 2:w249:dbl)
                n80 = Multiply(x=w236, y=0.001) -> (x*y=w231:dbl)
                n81 = Negate(x=w220) -> (-x=w219:dbl)
                n82 = Index Array(array=w242, index=w240) -> (element=w241:dbl)
                n83 = Multiply(x=w243, y=w249) -> (x*y=w246:dbl[])
                n84 = Multiply(x=w241, y=w250) -> (x*y=w248:dbl)
                n85 = Multiply(x=w241, y=w249) -> (x*y=w245:dbl)
                n86 = Multiply(x=w243, y=w250) -> (x*y=w244:dbl[])
                n87 = Negate(x=w248) -> (-x=w247:dbl)
                n88 = Compound Arithmetic op=unknown(w244, w245, w218) -> (w232:dbl[])
                n89 = Compound Arithmetic op=unknown(w246, w247, w219) -> (w233:dbl[])
                n90 = Multiply(x=w233, y=w231) -> (x*y=w230:dbl[])
                n91 = Multiply(x=w232, y=w231) -> (x*y=w227:dbl[])
                n92 = Insert Into Array(array=w228, new element=w230) -> (w229:dbl[])  [unwired: 1 in]
                n93 = Insert Into Array(array=w226, new element=w227) -> (w225:dbl[])  [unwired: 1 in]
              }
              n94 = Bundle("Value"=w182, "Value"=w181) -> (w180:cluster{"Value":u32, "Value":u32})  [unwired: 1 in]
              n95 = Divide(x=w180, y=2) -> (x/y=w184:cluster{"Value":dbl, "Value":dbl})
              n96 = property on="Channel2" class="IntensityGraph (strict)"("Cursor.Cursor Position"=w184) -> ()  [unwired: 2 in, 2 out]
              n97 = Array Size(array=w206) -> (size(s)=w207:i32)
              n98 = Bundle By Name(cluster=cluster{"Fs":dbl, "#s":dbl} {"Fs"=1000.0, "#s"=1000.0} ("sampling info"), "Fs"=w207, "#s"=w207) -> (w212:cluster{"Fs":dbl, "#s":dbl})
              n99 = Array Size(array=w189) -> (size(s)=w201:i32)
              n100 = Index Array(array=w189, index=0) -> (element=w193:dbl)
              n101 = Array Size(array=w188) -> (size(s)=w204:i32)
              n102 = Index Array(array=w188, index=0) -> (element=w198:dbl)
              n103 = Decrement(x=w201) -> (x-1=w200:i32)
              n104 = Index Array(array=w189, index=w200) -> (element=w192:dbl)
              n105 = call <vilib>:"Basic Function Generator.vi"("offset"=w208, "sampling info"=w212, "signal type"=T1."Sawtooth Wave", "phase"=180.0, "amplitude"=w208, "frequency"=1.0) -> ("signal out"=w210:waveform(dbl))  [unwired: 3 in, 2 out]
              n106 = Decrement(x=w204) -> (x-1=w203:i32)
              n107 = Index Array(array=w188, index=w203) -> (element=w196:dbl)
              n108 = Subtract(x=w198, y=w196) -> (x-y=w199:dbl)
              n109 = Unbundle By Name(w210) -> ("Y"=w191:dbl[])
              n110 = Subtract(x=w193, y=w192) -> (x-y=w195:dbl)
              n111 = Multiply(x=w199, y=w191) -> (x*y=w197:dbl[])
              n112 = Multiply(x=w195, y=w191) -> (x*y=w194:dbl[])
              n113 = Add(x=w197, y=w196) -> (x+y=w190:dbl[])
              n114 = Add(x=w194, y=w192) -> (x+y=w185:dbl[])
              n115 = Insert Into Array(array=w188, new element=w190) -> (w187:dbl[])  [unwired: 1 in]
              n116 = Insert Into Array(array=w189, new element=w185) -> (w186:dbl[])  [unwired: 1 in]
              n117 = Build Array(w187, w186) -> (w179:dbl[][])
            }
            frame #3 {
              w285 = 0.5 ("offset")
              # "Move to the initial point"
              # "current position"
              n118 = Array Size(array=w265) -> (size(s)=w264:i32)
              n119 = Bundle By Name(cluster=cluster{"Fs":dbl, "#s":dbl} {"Fs"=1000.0, "#s"=1000.0} ("sampling info"), "Fs"=w264, "#s"=w264) -> (w289:cluster{"Fs":dbl, "#s":dbl})
              n120 = call-poly <vilib>:"DAQmx Create Virtual Channel.vi"("maximum value"=10.0 ("Maximum Value 2"), "minimum value"=-10.0 ("Minimum Value 2"), "physical channels"="Starting Point for Scan") -> ("task out"=w295:refnum<k21>, "error out"=w294:errorcluster)  [unwired: 11 in]
              n121 = call <vilib>:"Basic Function Generator.vi"("offset"=w285, "sampling info"=w289, "signal type"=T1."Sawtooth Wave", "phase"=180.0, "amplitude"=w285, "frequency"=1.0) -> ("signal out"=w287:waveform(dbl))  [unwired: 3 in, 2 out]
              n122 = Index Array(array=w261, index (col)=0 ("disabled index (col)")) -> (element=w281:dbl[])  [unwired: 1 in]
              n123 = Unbundle By Name(w287) -> ("Y"=w267:dbl[])
              n124 = call-poly <vilib>:"DAQmx Read.vi"("task/channels in"=w295, "timeout"=10.0, "error in"=w294) -> ("data"=w283:dbl[])  [unwired: 10 in, 2 out]
              n125 = Index Array(array=w281, index=0) -> (element=w278:dbl)
              n126 = Index Array(array=w281, index=1) -> (element=w273:dbl)
              n127 = Index Array(array=w283, index=0) -> (element=w277:dbl)
              n128 = Index Array(array=w283, index=1) -> (element=w274:dbl)
              n129 = Subtract(x=w273, y=w274) -> (x-y=w272:dbl)
              n130 = Subtract(x=w278, y=w277) -> (x-y=w276:dbl)
              n131 = Multiply(x=w276, y=w267) -> (x*y=w275:dbl[])
              n132 = Multiply(x=w272, y=w267) -> (x*y=w271:dbl[])
              n133 = Add(x=w277, y=w275) -> (x+y=w270:dbl[])
              n134 = Add(x=w274, y=w271) -> (x+y=w269:dbl[])
              n135 = Divide(x=w256, y=2) -> (x/y=w259:dbl)
              n136 = Divide(x=w255, y=2) -> (x/y=w257:dbl)
              n137 = Build Array(w270, w269) -> (w262:dbl[][])
              n138 = property on="Channel2" class="IntensityGraph (strict)"("Cursor.Cursor Position:Cursor Y"=w257) -> ()  [unwired: 2 in, 2 out]
              n139 = property on="Channel2" class="IntensityGraph (strict)"("Cursor.Cursor Position:Cursor X"=w259) -> ()  [unwired: 2 in, 2 out]
              n140 = call-poly <vilib>:"DAQmx Write.vi"("task/channels in"=w263, "auto start"=TRUE, "data"=w262) -> ("task out"=w266:refnum<k21>)  [unwired: 10 in, 2 out]
              n141 = call <vilib>:"DAQmx Stop Task.vi"("task/channels in"=w266) -> ()  [unwired: 13 in, 2 out]
            }
            frame #4 {
              n142 = while {
                tunnel: w319 -> [w369]
                tunnel: w318 -> [w368]
                tunnel: w317 -> [w322]
                tunnel: [w350] -> w316
                tunnel: [w349] -> w315
                tunnel: [w347] -> w314
                tunnel: [w346] -> w313
                tunnel: [w345] -> w312
                tunnel: w311 -> [w344]
                tunnel: [w343] -> w310
                tunnel: w309 -> [w342]
                tunnel: w308 -> [w341]
                tunnel: w307 -> [w321]
                tunnel: [w340] -> w306
                tunnel: [w339] -> w305
                tunnel: w304 -> [w336]
                tunnel: [w335] -> w303
                tunnel: w302 -> [w334]
                tunnel: w301 -> [w332]
                tunnel: [w330] -> w300
                tunnel: [w329] -> w299
                stop <- w326 stop-if-true
                n143 = property class="DAQmx Timing"(reference=w369, error in=w368) -> (reference out=w367:refnum<k21>, error out=w366:errorcluster, "Sample Clock:Rate"=→"Input rate":dbl)
                n144 = property class="DAQmx Timing"(reference=w321, error in=w322) -> (reference out=w323:refnum<k21>, error out=w363:errorcluster, "Sample Clock:Rate"=→"Output rate":dbl)
                n145 = call "Get Terminal Name with Device Prefix.vi"("error in (no error)"=w366, "Local Terminal Name"="ai/StartTrigger" ("terminal"), "task/channels in"=w367) -> ("error out"=w356:errorcluster, "Terminal Name with Device Prefix"=w364:tag, "task out"=w357:refnum<k21>)  [unwired: 6 in]
                n146 = call-poly <vilib>:"DAQmx Trigger.vi"("task/channels in"=w323, "source"=w364, "error in"=w363) -> ("task out"=w362:refnum<k21>, "error out"=w361:errorcluster)  [unwired: 11 in]
                n147 = call-poly <vilib>:"DAQmx Write.vi"("task/channels in"=w362, "data"=w341, "timeout"=10.0 ("Wirite Timeout"), "error in"=w361) -> ("task out"=w359:refnum<k21>, "error out"=w358:errorcluster)  [unwired: 9 in, 1 out]
                n148 = call <vilib>:"DAQmx Start Task.vi"("task/channels in"=w359, "error in"=w358) -> ("task out"=w338:refnum<k21>, "error out"=w355:errorcluster)  [unwired: 12 in]
                n149 = call <vilib>:"Merge Errors.vi"("error in 2 (no error)"=w355, "error in 1 (no error)"=w356) -> ("error out"=w354:errorcluster)  [unwired: 5 in]
                n150 = call <vilib>:"DAQmx Start Task.vi"("task/channels in"=w357, "error in"=w354) -> ("task out"=w337:refnum<k21>, "error out"=w353:errorcluster)  [unwired: 12 in]
                n151 = Unbundle By Name(w336) -> ("Continuous \nScan"=w348:bool)
                n152 = call <vilib>:"DAQmx Start Task.vi"("task/channels in"=w334, "error in"=w332) -> ("task out"=w325:refnum<k21>, "error out"=w333:errorcluster)  [unwired: 12 in]
                n153 = while {
                  tunnel: w337 -> [w420]
                  tunnel: w353 -> [w419]
                  tunnel: w338 -> [w409]
                  tunnel: w342 -> [w411]
                  tunnel: w336 -> [w407]
                  tunnel: [w415] -> w352
                  shift-right: [w398] -> _
                  shift-left: w344 -> [w412]
                  tunnel: ["Stop"] -> w350
                  shift-right: [w397] -> _
                  shift-left: w344 -> [w404]
                  tunnel: [w398] -> w340
                  tunnel: [w397] -> w339
                  tunnel: ["Reset"] -> w335
                  tunnel: w325 -> [w395]
                  tunnel: w333 -> [w394]
                  tunnel: [w393] -> w331
                  tunnel: ["Reset"] -> w328
                  tunnel: ["Stop"] -> w320
                  tunnel: ["?"] -> w327
                  tunnel: [w383] -> _
                  i -> [w392]
                  stop <- w421 stop-if-true
                  n154 = Unbundle By Name(w407) -> ("Scan Rate (Hz)"=w405:dbl, "Scan Lines"=w387:u32, "Continuous \nScan"=w406:bool, "Scan Points"=w401:u32, "Lines read"=w391:u32, "Scanner delay (ms)"=w403:dbl)
                  n155 = Quotient & Remainder(x=w411, y=w405) -> (floor(x/y)=w408:dbl)  [unwired: 1 out]
                  n156 = Multiply(x=w408, y=w391) -> (x*y=w399:dbl)
                  n157 = call-poly <vilib>:"DAQmx Read.vi"("task/channels in"=w420, "number of samples per channel"=w399, "error in"=w419) -> ("data"=w390:dbl[][], "error out"=w418:errorcluster)  [unwired: 10 in, 1 out]
                  n158 = call <vilib>:"DAQmx Is Task Done.vi"("task/channels in"=w409, "error in"=w418) -> ("task out"=w383:refnum<k21>, "error out"=w417:errorcluster)  [unwired: 11 in, 1 out]
                  n159 = Unbundle By Name(w417) -> ("status"=w416:bool)
                  n160 = call <vilib>:"DAQmx Is Read or Write Late.vi"("error in"=w417) -> ("error out"=w415:errorcluster)  [unwired: 13 in, 1 out]
                  n161 = Quotient & Remainder(x=w387, y=w391) -> (floor(x/y)=w400:u32)  [unwired: 1 out]
                  n162 = Compound Arithmetic op=MULTIPLY(w403, w411, 0.001 ("value")) -> (w380:dbl)
                  n163 = Greater Or Equal?(x=w392, y=w400) -> (x >= y?=w414:bool)
                  n164 = stacked-sequence {
                    seq-local: [w457 _] -> [_ w549]
                    tunnel: w412 -> [w464 w550]
                    tunnel: [w454 _] -> w398
                    tunnel: w380 -> [w463 _]
                    tunnel: w392 -> [w462 _]
                    tunnel: w401 -> [w461 _]
                    tunnel: w408 -> [w460 _]
                    tunnel: w387 -> [w456 _]
                    tunnel: w390 -> [w459 _]
                    tunnel: w391 -> [w453 _]
                    tunnel: w404 -> [w458 w544]
                    tunnel: [w455 _] -> w397
                    tunnel: [_ w545] -> w402
                    frame #0 {
                      n165 = while {
                        tunnel: w459 -> [w490]
                        tunnel: w462 -> [w474]
                        tunnel: w456 -> [w478]
                        tunnel: w460 -> [w485]
                        tunnel: w461 -> [w482]
                        tunnel: w453 -> [w475]
                        shift-right: [w488] -> w454
                        shift-left: w464 -> [w489]
                        tunnel: w463 -> [w470]
                        tunnel: [w465] -> w452
                        i -> [w472]
                        stop <- w480 stop-if-true
                        n166 = Decrement(x=w475) -> (x-1=w481:u32)
                        n167 = Index Array(array=w490, index (row)=0) -> (element=w487:dbl[])  [unwired: 1 in]
                        n168 = Multiply(x=w474, y=w475) -> (x*y=w476:u32)
                        n169 = Add(x=0.26666 ("value"), y=w472) -> (x+y=w468:dbl)
                        n170 = Greater Or Equal?(x=w472, y=w481) -> (x >= y?=w480:bool)
                        n171 = Add(x=w476, y=w472) -> (x+y=w477:u32)
                        n172 = Compound Arithmetic op=MULTIPLY(w468, w485) -> (w471:dbl)
                        n173 = Quotient & Remainder(x=w477, y=w478) -> (x-y*floor(x/y)=w479:u32)  [unwired: 1 out]
                        n174 = Add(x=w470, y=w471) -> (x+y=w469:dbl)
                        n175 = Negate(x=w469) -> (-x=w467:dbl)
                        n176 = Round To Nearest(number=w467) -> (nearest integer value=w486:dbl)
                        n177 = Rotate 1D Array(1:w487, 2:w486) -> (0:w466:dbl[])
                        n178 = Initialize Array(0.0 ("element"), w482) -> (w484:dbl[])
                        n179 = while {
                          tunnel: w466 -> [w500]
                          tunnel: w482 -> [w497]
                          tunnel: w485 -> [w502]
                          shift-right: [w495] -> w465
                          shift-left: w484 -> [w494]
                          i -> [w492]
                          stop <- w498 stop-if-true
                          n180 = Decrement(x=w497) -> (x-1=w496:u32)
                          n181 = Greater Or Equal?(x=w492, y=w496) -> (x >= y?=w498:bool)
                          n182 = Compound Arithmetic op=MULTIPLY(0.6666 ("value"), w502, w492) -> (w501:dbl)
                          n183 = Quotient & Remainder(x=w501, y=w497) -> (floor(x/y)=w499:dbl)  [unwired: 1 out]
                          n184 = Index Array(array=w500, index=w499) -> (element=w493:dbl)
                          n185 = Replace Array Subset(array=w494, new element=w493, index=w492) -> (w495:dbl[])
                        }
                        n186 = Replace Array Subset(array=w489, new element=w465, index (col)=w479) -> (w488:dbl[][])  [unwired: 1 in]
                      }
                      "Reflection Image" <- w454
                      n187 = while {
                        tunnel: w459 -> [w529]
                        tunnel: w462 -> [w516]
                        tunnel: w456 -> [w519]
                        tunnel: w460 -> [w524]
                        tunnel: w461 -> [w521]
                        tunnel: w453 -> [w506]
                        shift-right: [w527] -> w455
                        shift-left: w458 -> [w528]
                        tunnel: w463 -> [w513]
                        tunnel: [w505] -> w457
                        tunnel: [w504] -> w451
                        i -> [w507]
                        stop <- w508 stop-if-true
                        n188 = Decrement(x=w506) -> (x-1=w520:u32)
                        n189 = Index Array(array=w529, index (row)=1) -> (element=w526:dbl[])  [unwired: 1 in]
                        n190 = Multiply(x=w516, y=w506) -> (x*y=w517:u32)
                        n191 = Add(x=0.26666 ("value"), y=w507) -> (x+y=w511:dbl)
                        n192 = Greater Or Equal?(x=w507, y=w520) -> (x >= y?=w508:bool)
                        n193 = Add(x=w517, y=w507) -> (x+y=w518:u32)
                        n194 = Compound Arithmetic op=MULTIPLY(w511, w524) -> (w514:dbl)
                        n195 = Quotient & Remainder(x=w518, y=w519) -> (x-y*floor(x/y)=w505:u32)  [unwired: 1 out]
                        n196 = Add(x=w513, y=w514) -> (x+y=w512:dbl)
                        n197 = Negate(x=w512) -> (-x=w510:dbl)
                        n198 = Round To Nearest(number=w510) -> (nearest integer value=w525:dbl)
                        n199 = Rotate 1D Array(1:w526, 2:w525) -> (0:w509:dbl[])
                        n200 = Initialize Array(0.0 ("element"), w521) -> (w523:dbl[])
                        n201 = while {
                          tunnel: w509 -> [w539]
                          tunnel: w521 -> [w536]
                          tunnel: w524 -> [w541]
                          shift-right: [w534] -> w504
                          shift-left: w523 -> [w533]
                          i -> [w531]
                          stop <- w537 stop-if-true
                          n202 = Decrement(x=w536) -> (x-1=w535:u32)
                          n203 = Greater Or Equal?(x=w531, y=w535) -> (x >= y?=w537:bool)
                          n204 = Compound Arithmetic op=MULTIPLY(0.6666 ("value"), w541, w531) -> (w540:dbl)
                          n205 = Quotient & Remainder(x=w540, y=w536) -> (floor(x/y)=w538:dbl)  [unwired: 1 out]
                          n206 = Index Array(array=w539, index=w538) -> (element=w532:dbl)
                          n207 = Replace Array Subset(array=w533, new element=w532, index=w531) -> (w534:dbl[])
                        }
                        n208 = Replace Array Subset(array=w528, new element=w504, index (col)=w505) -> (w527:dbl[][])  [unwired: 1 in]
                      }
                      "Channel2" <- w455
                      n209 = Build Array(w452, w451) -> (→"Linescan":dbl[][])
                    }
                    frame #1 {
                      n210 = property on="Scan Lines" class="Digital (strict)"() -> ("Value"=w547:u32)  [unwired: 2 in, 2 out]
                      n211 = Decrement(x=w547) -> (x-1=w546:u32)
                      n212 = Equal?(x=w546, y=w549) -> (x = y?=w548:bool)
                      n213 = And(x="Save Image", y=w548) -> (x .and. y?=w545:bool)
                      n214 = case shown="True" w545 {
                        tunnel: w550 -> [_ w564]
                        tunnel: w544 -> [_ w563]
                        frame #0 {
                        }
                        frame #1 {
                          w566 = "%.3f" ("format string")
                          w569 = T3."create or replace" ("function (open:0)")
                          n215 = case shown="True" "Concat" {
                            tunnel: [w579 w582] -> w557
                            tunnel: "Channel 2" -> [w579 w583]
                            tunnel: [w578 w589] -> w555
                            tunnel: "Channel 1" -> [w578 w594]
                            frame #0 {
                            }
                            frame #1 {
                              w581 = "_"
                              n216 = local read "Output3"() -> (w591:dbl)
                              n217 = Multiply(x=w591, y=1000) -> (x*y=w590:dbl)
                              n218 = Strip Path(path=w594) -> (stripped path=w588:path, name=w593:string)
                              n219 = Strip Path(path=w583) -> (stripped path=w585:path, name=w586:string)
                              n220 = Number To Decimal String(number=w590) -> (decimal integer string=w580:string)  [unwired: 1 in]
                              n221 = Concatenate Strings(w593, w581, w580) -> (w587:string)
                              n222 = Concatenate Strings(w586, w581, w580) -> (w584:string)
                              n223 = Build Path(base path=w588, name or relative path=w587) -> (appended path=w589:path)
                              n224 = Build Path(base path=w585, name or relative path=w584) -> (appended path=w582:path)
                            }
                          }
                          n225 = call <vilib>:"Open_Create_Replace File.vi"("function (open:0)"=w569, "file path"=w555) -> ("error out"=w575:errorcluster, "refnum"=w577:refnum<file>)  [unwired: 6 in, 2 out]
                          n226 = call <vilib>:"Open_Create_Replace File.vi"("function (open:0)"=w569, "file path"=w557) -> ("error out"=w573:errorcluster, "refnum"=w572:refnum<file>)  [unwired: 6 in, 2 out]
                          n227 = Array To Spreadsheet String(array=w563, 3:w566) -> (spreadsheet string=w567:string)  [unwired: 1 in]
                          n228 = Array To Spreadsheet String(array=w564, 3:w566) -> (spreadsheet string=w568:string)  [unwired: 1 in]
                          n229 = Write to Binary File(file (use dialog)=w572, data=w567, error in=w573, 5:FALSE ("prepend array or string size? (T)")) -> (refnum out=w571:refnum<file>, error out=w570:errorcluster)  [unwired: 2 in, 1 out]
                          n230 = Write to Binary File(file (use dialog)=w577, data=w568, error in=w575, 5:FALSE ("prepend array or string size? (T)")) -> (refnum out=w576:refnum<file>, error out=w574:errorcluster)  [unwired: 2 in, 1 out]
                          n231 = property on="Increment" class="Bool (strict)"() -> ("Value"=w558:bool)  [unwired: 2 in, 2 out]
                          n232 = Close File(refnum=w576, error in=w574) -> (error out=w565:errorcluster)  [unwired: 1 out]
                          n233 = Close File(refnum=w571, error in=w570) -> (error out=w561:errorcluster)  [unwired: 1 out]
                          n234 = call <vilib>:"Merge Errors.vi"("error in 2 (no error)"=w561, "error in 1 (no error)"=w565) -> ("error out"=w562:errorcluster)  [unwired: 5 in]
                          n235 = call <vilib>:"Simple Error Handler.vi"("error in (no error)"=w562) -> ("error?"=w559:bool)  [unwired: 4 in, 4 out]
                          n236 = Or(x=w559, y=w558) -> (x .or. y?=w560:bool)
                          n237 = local write "Save Image"(w560) -> ()
                        }
                      }
                    }
                  }
                  n238 = Not(x=w406) -> (.not. x?=w413:bool)
                  n239 = And(x=w414, y=w413) -> (x .and. y?=w396:bool)
                  n240 = Multiply(x=w392, y=w391) -> (x*y=w388:u32)
                  n241 = Divide(x=w388, y=w387) -> (x/y=w386:dbl)
                  n242 = Quotient & Remainder(x=w388, y=w387) -> (floor(x/y)=w389:u32)  [unwired: 1 out]
                  n243 = Equal?(x=w389, y=w386) -> (x = y?=w382:bool)
                  n244 = And(x="Increment", y=w382) -> (x .and. y?=w376:bool)
                  n245 = case shown="True" w376 {
                    tunnel: "Output3" -> [w436 w437]
                    tunnel: [w436 w438] -> w375
                    frame #0 {
                    }
                    frame #1 {
                      n246 = Greater?(x="stepsize", y=0) -> (0:w442:bool)
                      n247 = Less?(x=w437, y="StopPoint") -> (x < y?=w441:bool)
                      n248 = Exclusive Or(1:w441, 2:w442) -> (0:w440:bool)
                      n249 = case shown="False" w440 {
                        tunnel: "stepsize" -> [w447 _]
                        tunnel: w437 -> [w446 w448]
                        tunnel: [w445 w448] -> w438
                        frame #0 {
                          n250 = Add(x=w446, y=w447) -> (x+y=w445:dbl)
                        }
                        frame #1 {
                          n251 = local write "Increment"(FALSE) -> ()
                        }
                      }
                    }
                  }
                  n252 = event shown="[2] \"Channel2\": Mouse Enter" {
                    selector: _ -> [_ _ _]
                    dyn-events: _ -> [_ _ _]
                    timeout: 0 -> [_ _ _]
                    tunnel: [w422 TRUE FALSE] -> w374
                    event #0 {
                      n253 = event-data() -> ()  [unwired: 1 in, 2 out]
                      n254 = local read "Boolean"() -> (w422:bool)
                    }
                    event #1 {
                      n255 = event-data() -> ()  [unwired: 1 in, 4 out]
                    }
                    event #2 {
                      n256 = event-data() -> ()  [unwired: 1 in, 4 out]
                    }
                  }
                  "Boolean" <- w374
                  n257 = Compound Arithmetic op=OR(w396, "Reset", "Stop", w416, w402, "?", "?") -> (w421:bool)
                  n258 = case shown="False" w374 {
                    frame #0 {
                      n259 = property on="Channel2" class="IntensityGraph (strict)"() -> ("Cursor.Cursor Position"=w425:T4)  [unwired: 2 in, 2 out]
                      n260 = property on="Reflection Image" class="IntensityGraph (strict)"("Cursor.Cursor Position"=w425) -> ()  [unwired: 2 in, 2 out]
                    }
                    frame #1 {
                      n261 = property on="Reflection Image" class="IntensityGraph (strict)"() -> ("Cursor.Cursor Position"=w426:T4)  [unwired: 2 in, 2 out]
                      n262 = property on="Channel2" class="IntensityGraph (strict)"("Cursor.Cursor Position"=w426) -> ()  [unwired: 2 in, 2 out]
                    }
                  }
                  n263 = local write "Output3"(w375) -> ()
                  n264 = Or(x=w376, y="Update") -> (x .or. y?=w378:bool)
                  n265 = case shown="True" w378 {
                    tunnel: w395 -> [_ w435]
                    tunnel: w394 -> [w427 w432]
                    tunnel: [w427 w431] -> w393
                    tunnel: w375 -> [_ w429]
                    frame #0 {
                    }
                    frame #1 {
                      n266 = Bundle("Output3"=w429, "Output4"="Output4") -> (w433:cluster{"Output3":dbl, "Output4":dbl})  [unwired: 1 in]
                      n267 = local write "Update"(FALSE ("Update")) -> ()
                      n268 = Cluster To Array(cluster=w433) -> (array=w434:dbl[])
                      n269 = call-poly <vilib>:"DAQmx Write.vi"("task/channels in"=w435, "data"=w434, "error in"=w432) -> ("error out"=w431:errorcluster)  [unwired: 10 in, 2 out]
                    }
                  }
                }
                n270 = Not(x=w348) -> (.not. x?=w343:bool)
                n271 = call <vilib>:"DAQmx Stop Task.vi"("task/channels in"=w338, "error in"=w352) -> ("task out"=w345:refnum<k21>, "error out"=w351:errorcluster)  [unwired: 12 in]
                n272 = call <vilib>:"DAQmx Stop Task.vi"("task/channels in"=w337, "error in"=w351) -> ("task out"=w347:refnum<k21>, "error out"=w346:errorcluster)  [unwired: 12 in]
                n273 = Unbundle By Name(w346) -> ("status"=w349:bool)
                n274 = case shown="False" w327 {
                  frame #0 {
                  }
                  frame #1 {
                    n275 = while {
                      stop <- w371 continue-if-true
                      n276 = property class="Boolean (strict)"() -> ("Value"=w371:bool)  [unwired: 2 in, 2 out]
                    }
                  }
                }
                n277 = call <vilib>:"DAQmx Stop Task.vi"("task/channels in"=w325, "error in"=w331) -> ("task out"=w329:refnum<k21>, "error out"=w330:errorcluster)  [unwired: 12 in]
                n278 = Compound Arithmetic op=OR(w328, w320) -> (w326:bool)
              }
            }
            frame #5 {
              n279 = property on="Channel2" class="IntensityGraph (strict)"() -> ("Cursor.Cursor Position"=w600:T4)  [unwired: 2 in, 2 out]
              n280 = Bundle("Value"=w595, "Value"=w596) -> (w615:cluster{"Value":u32, "Value":u32})  [unwired: 1 in]
              n281 = Unbundle By Name(w621) -> ("Scan Angle (degrees)"=w624:dbl)
              n282 = Reciprocal(x=180.0 ("value")) -> (1/x=w622:dbl)
              n283 = Divide(x=w615, y=2) -> (x/y=w620:cluster{"Value":dbl, "Value":dbl})
              n284 = Compound Arithmetic op=MULTIPLY(w624, w622, 3.141592653589793) -> (w625:dbl)
              n285 = Subtract(x=w600, y=w620) -> (x-y=w616:T4)
              n286 = Sine & Cosine(0:w625) -> (1:w619:dbl, 2:w618:dbl)
              n287 = Divide(x=w616, y=w615) -> (x/y=w617:T4)
              n288 = Negate(x=w619) -> (-x=w597:dbl)
              n289 = Multiply(x=w597, y=w617) -> (x*y=w613:T4)
              n290 = Multiply(x=w618, y=w617) -> (x*y=w614:T4)
              n291 = Unbundle(w614) -> ("Cursor X"=w612:dbl, "Cursor Y"=w610:dbl)
              n292 = Unbundle(w613) -> ("Cursor X"=w609:dbl, "Cursor Y"=w611:dbl)
              n293 = property on="Y Scan size(um)" class="Digital (strict)"() -> ("Value"=w606:dbl)  [unwired: 2 in, 2 out]
              n294 = Negate(x=w609) -> (-x=w608:dbl)
              n295 = Add(x=w611, y=w612) -> (x+y=w601:dbl)
              n296 = Add(x=w608, y=w610) -> (x+y=w599:dbl)
              n297 = property on="X Scan size(um)" class="Digital (strict)"() -> ("Value"=w607:dbl)  [unwired: 2 in, 2 out]
              n298 = Negate(x=w606) -> (-x=w598:dbl)
              n299 = Bundle(w601, w599) -> (w605:cluster{dbl, dbl})  [unwired: 1 in]
              n300 = Bundle("Value"=w607, w598) -> (w604:cluster{"Value":dbl, dbl})  [unwired: 1 in]
              n301 = Multiply(x=w605, y=w604) -> (x*y=w602:cluster{dbl, dbl})
              n302 = flat-sequence {
                tunnel: [w630] -> w603
                tunnel: w603 -> [w635]
                tunnel: w602 -> [w634]
                frame #0 {
                  n303 = local read "Y offset (um)"() -> (w628:dbl)
                  n304 = local read "X offset (um)"() -> (w629:dbl)
                  n305 = Bundle("X offset (um)"=w629, "Y offset (um)"=w628) -> (w630:T5)  [unwired: 1 in]
                }
                frame #1 {
                  n306 = Subtract(x=w635, y=w634) -> (x-y=w633:cluster{dbl, dbl})
                  n307 = Unbundle(w633) -> (w632:dbl, w631:dbl)
                  n308 = local write "Y offset (um)"(w631) -> ()
                  n309 = local write "X offset (um)"(w632) -> ()
                }
              }
            }
          }
          n310 = Compound Arithmetic op=OR(w77, w81, w89, w76) -> (w86:bool)
        }
        n311 = call <vilib>:"DAQmx Clear Task.vi"("task in"=w52, "error in"=w53) -> ()  [unwired: 13 in, 1 out]
        n312 = call <vilib>:"DAQmx Clear Task.vi"("task in"=w66, "error in"=w65) -> ("error out"=w54:errorcluster)  [unwired: 13 in]
        n313 = call <vilib>:"DAQmx Clear Task.vi"("task in"=w64, "error in"=w54) -> ("error out"=w63:errorcluster)  [unwired: 13 in]
        n314 = call <vilib>:"General Error Handler.vi"("error in (no error)"=w63) -> ()  [unwired: 10 in, 5 out]
      }
    }
  }
